vi "Dunk Tank Cal UI.vi"(11 "Calling VI Ref":refnum<vi>) -> ()   [LabVIEW 2013]
uses:
  Netway Driver/Type Defs/Communication Function Type Def.ctl
  <vilib>/ptbypt/NI_PtbyPt.lvlib
  <vilib>/Utility/file.llb/Read From Spreadsheet File (string).vi
  <vilib>/Utility/miscctls.llb/LVRowAndColumnTypeDef.ctl
  <vilib>/Analysis/NI_AALPro.lvlib
  <resource>/objmgr/daqmx.rc
  <vilib>/Utility/file.llb/Write To Spreadsheet File (string).vi
panel:
  in  "App Dir":path
  in  "Load Indicator Tab":enum32{"Page 1"}(tab)
  in  "Header Tab":enum32{"Page 1", "Page 2"}(tab)
  in  "Header OK":bool
  in  "Header Cancel":bool
  in  "Header Comments":string[][](table)=[["PRODUCT 5V. IS REFERENCE ONLY."], ["1"], ["2"]]
  in  "Cal Standards Table":string[][](table)=[["FLUKE MULTIMETER", "3539"], ["FLUKE CALIBRATOR", "7955"], ["", ""], ["", ""], ["", ""]]
  in  "Sys Cal Table":string[][](table)=[["CIB BD.", "DSS 9372-1"], ["D/A BD.", "DSS 9372-2"], ["", ""], ["", ""], ["", ""]]
  in  "Header Table 1":string[][](table)=[["9372blah"], ["DELPHI"], ["TL1181E"], ["EU2C397"], ["CIB/ D/A BD."], ["5 VOLTS"], ["NEW"], ["9087"]]
  in  "Header Table 2":string[][](table)=[["39687"], ["12"], ["40052"], ["MDC"], ["24"], ["48"], ["JUM  /   DR"]]
  in  "debug":bool=TRUE
  in  "Verify Tab":enum32{"Page 1", "Page 2"}(tab)
  in  "Hide Devs":bool
  in  "Auto":bool
  in  "Hide Cal Values":bool
  in  "Verify Edit":bool
  in  "Verify Table":string[][](table)=[["", "0", "0"], ["", "3", "3"], ["", "6", "6"], ["", "9", "9"], ["", "12", "12"], ["", "15", "15"], ["", "", ""], ["", "", ""], ["", "", ""], ["", "", ""]]
  in  "Verify Read":bool
  in  "ms":u32=1000
  in  "avg":i32=5
  in  "Output Tab":enum32{"Page 1", "Page 2"}(tab)
  in  "Close Outputs":bool
  in  "Output Question":bool
  in  "Set Output Next":bool
  in  "Set Output":bool
  in  "Output Listbox":i32(listbox)
  out "Row":i32
  in  "Main Tab":enum32{"Page 1", "Page 2"}(tab)
  in  "View Spreadsheet":bool
  in  "Header":bool
  out "Cal Table":string[][](table)=[["AI-00", "V", "", "", "", "", "", "", "", "", "", "", "", "", "", "", "", "", "", "", "", "", "", "", "", "", "", "", "", "", "", ""], ["AI-01", "V", "", "", "", "", "", "", "", "", "", "", "", "", "", "", "", "", "", "", "", "", "", "", "", "", "", "", "", "", "", ""], ["AI-02", "V", "", "", "", "", "", "", "", "", "", "", "", "", "", "", "", "", "", "", "", "", "", "", "", "", "", "", "", "", "", ""], ["AI-03", "V", "", "", "", "", "", "", "", "", "", "", "", "", "", "", "", "", "", "", "", "", "", "", "", "", "", "", "", "", "", ""], ["AI-04", "V", "", "", "", "", "", "", "", "", "", "", "", "", "", "", "", "", "", "", "", "", "", "", "", "", "", "", "", "", "", ""], ["AI-05", "V", "", "", "", "", "", "", "", "", "", "", "", "", "", "", "", "", "", "", "", "", "", "", "", "", "", "", "", "", "", ""], ["AI-06", "V", "", "", "", "", "", "", "", "", "", "", "", "", "", "", "", "", "", "", "", "", "", "", "", "", "", "", "", "", "", ""], ["AI-07", "V", "", "", "", "", "", "", "", "", "", "", "", "", "", "", "", "", "", "", "", "", "", "", "", "", "", "", "", "", "", ""], ["AI-08", "V", "", "", "", "", "", "", "", "", "", "", "", "", "", "", "", "", "", "", "", "", "", "", "", "", "", "", "", "", "", ""], ["AI-09", "V", "", "", "", "", "", "", "", "", "", "", "", "", "", "", "", "", "", "", "", "", "", "", "", "", "", "", "", "", "", ""], ["AI-10", "V", "", "", "", "", "", "", "", "", "", "", "", "", "", "", "", "", "", "", "", "", "", "", "", "", "", "", "", "", "", ""], ["AI-11", "V", "", "", "", "", "", "", "", "", "", "", "", "", "", "", "", "", "", "", "", "", "", "", "", "", "", "", "", "", "", ""], ["AI-12", "V", "", "", "", "", "", "", "", "", "", "", "", "", "", "", "", "", "", "", "", "", "", "", "", "", "", "", "", "", "", ""], ["AI-13", "V", "", "", "", "", "", "", "", "", "", "", "", "", "", "", "", "", "", "", "", "", "", "", "", "", "", "", "", "", "", ""], ["AI-14", "V", "", "", "", "", "", "", "", "", "", "", "", "", "", "", "", "", "", "", "", "", "", "", "", "", "", "", "", "", "", ""], ["AI-15", "V", "", "", "", "", "", "", "", "", "", "", "", "", "", "", "", "", "", "", "", "", "", "", "", "", "", "", "", "", "", ""], ["AI-16", "V", "", "", "", "", "", "", "", "", "", "", "", "", "", "", "", "", "", "", "", "", "", "", "", "", "", "", "", "", "", ""], ["AI-17", "V", "", "", "", "", "", "", "", "", "", "", "", "", "", "", "", "", "", "", "", "", "", "", "", "", "", "", "", "", "", ""], ["AI-18", "V", "", "", "", "", "", "", "", "", "", "", "", "", "", "", "", "", "", "", "", "", "", "", "", "", "", "", "", "", "", ""], ["AI-19", "V", "", "", "", "", "", "", "", "", "", "", "", "", "", "", "", "", "", "", "", "", "", "", "", "", "", "", "", "", "", ""], ["AI-20", "V", "", "", "", "", "", "", "", "", "", "", "", "", "", "", "", "", "", "", "", "", "", "", "", "", "", "", "", "", "", ""], ["AI-21", "V", "", "", "", "", "", "", "", "", "", "", "", "", "", "", "", "", "", "", "", "", "", "", "", "", "", "", "", "", "", ""], ["AI-22", "V", "", "", "", "", "", "", "", "", "", "", "", "", "", "", "", "", "", "", "", "", "", "", "", "", "", "", "", "", "", ""], ["AI-23", "V", "", "", "", "", "", "", "", "", "", "", "", "", "", "", "", "", "", "", "", "", "", "", "", "", "", "", "", "", "", ""], ["AI-24", "V", "", "", "", "", "", "", "", "", "", "", "", "", "", "", "", "", "", "", "", "", "", "", "", "", "", "", "", "", "", ""], ["AI-25", "V", "", "", "", "", "", "", "", "", "", "", "", "", "", "", "", "", "", "", "", "", "", "", "", "", "", "", "", "", "", ""], ["AI-26", "V", "", "", "", "", "", "", "", "", "", "", "", "", "", "", "", "", "", "", "", "", "", "", "", "", "", "", "", "", "", ""], ["AI-27", "V", "", "", "", "", "", "", "", "", "", "", "", "", "", "", "", "", "", "", "", "", "", "", "", "", "", "", "", "", "", ""], ["AI-28", "V", "", "", "", "", "", "", "", "", "", "", "", "", "", "", "", "", "", "", "", "", "", "", "", "", "", "", "", "", "", ""], ["AI-29", "V", "", "", "", "", "", "", "", "", "", "", "", "", "", "", "", "", "", "", "", "", "", "", "", "", "", "", "", "", "", ""], ["AI-30", "V", "", "", "", "", "", "", "", "", "", "", "", "", "", "", "", "", "", "", "", "", "", "", "", "", "", "", "", "", "", ""], ["AI-31", "V", "", "", "", "", "", "", "", "", "", "", "", "", "", "", "", "", "", "", "", "", "", "", "", "", "", "", "", "", "", ""], ["TC-00", "degF", "", "", "", "", "", "", "", "", "", "", "", "", "", "", "", "", "", "", "", "", "", "", "", "", "", "", "", "", "", ""], ["TC-01", "degF", "", "", "", "", "", "", "", "", "", "", "", "", "", "", "", "", "", "", "", "", "", "", "", "", "", "", "", "", "", ""], ["TC-02", "degF", "", "", "", "", "", "", "", "", "", "", "", "", "", "", "", "", "", "", "", "", "", "", "", "", "", "", "", "", "", ""], ["TC-03", "degF", "", "", "", "", "", "", "", "", "", "", "", "", "", "", "", "", "", "", "", "", "", "", "", "", "", "", "", "", "", ""], ["TC-04", "degF", "", "", "", "", "", "", "", "", "", "", "", "", "", "", "", "", "", "", "", "", "", "", "", "", "", "", "", "", "", ""], ["TC-05", "degF", "", "", "", "", "", "", "", "", "", "", "", "", "", "", "", "", "", "", "", "", "", "", "", "", "", "", "", "", "", ""], ["TC-06", "degF", "", "", "", "", "", "", "", "", "", "", "", "", "", "", "", "", "", "", "", "", "", "", "", "", "", "", "", "", "", ""], ["TC-07", "degF", "", "", "", "", "", "", "", "", "", "", "", "", "", "", "", "", "", "", "", "", "", "", "", "", "", "", "", "", "", ""], ["TC-08", "degF", "", "", "", "", "", "", "", "", "", "", "", "", "", "", "", "", "", "", "", "", "", "", "", "", "", "", "", "", "", ""], ["TC-09", "degF", "", "", "", "", "", "", "", "", "", "", "", "", "", "", "", "", "", "", "", "", "", "", "", "", "", "", "", "", "", ""], ["TC-10", "degF", "", "", "", "", "", "", "", "", "", "", "", "", "", "", "", "", "", "", "", "", "", "", "", "", "", "", "", "", "", ""], ["TC-11", "degF", "", "", "", "", "", "", "", "", "", "", "", "", "", "", "", "", "", "", "", "", "", "", "", "", "", "", "", "", "", ""], ["TC-12", "degF", "", "", "", "", "", "", "", "", "", "", "", "", "", "", "", "", "", "", "", "", "", "", "", "", "", "", "", "", "", ""], ["TC-13", "degF", "", "", "", "", "", "", "", "", "", "", "", "", "", "", "", "", "", "", "", "", "", "", "", "", "", "", "", "", "", ""], ["TC-14", "degF", "", "", "", "", "", "", "", "", "", "", "", "", "", "", "", "", "", "", "", "", "", "", "", "", "", "", "", "", "", ""], ["TC-15", "degF", "", "", "", "", "", "", "", "", "", "", "", "", "", "", "", "", "", "", "", "", "", "", "", "", "", "", "", "", "", ""], ["", "", "", "", "", "", "", "", "", "", "", "", "", "", "", "", "", "", "", "", "", "", "", "", "", "", "", "", "", "", "", ""]]
  out "Dunk Tank":string
  in  "Channel to Cal":u16(ring) items=["AI-00", "AI-01", "AI-02", "AI-03", "AI-04", "AI-05", "AI-06", "AI-07", "AI-16", "AI-17", "AI-18", "AI-19", "AI-20", "AI-21", "AI-22", "AI-23"]
  in  "Start Cal":bool
  in  "Confirm 1st Point":bool
  out "Reading Value 1":dbl caption="reading" format="%#.4g"
  in  "Cal Value 1":dbl caption="cal pt" format="%#.4g"
  in  "Confirm 2nd Point":bool
  out "Reading Value 2":dbl=0.001 caption="reading" format="%#.4g"
  in  "Cal Value 2":dbl caption="cal pt" format="%#.4g"
  in  "Save Cal":bool
  out "f(x)":dbl format="%#.4g"
  out "a0":dbl format="%#.4g"
  out "x":dbl=0.0006000000000000001 format="%#.4g"
  out "a2":dbl format="%#.4g"
  in  "Cancel Cal":bool
  in  "Cal Unit":string
  in  "Confirm 3rd Point":bool
  out "Reading Value 3":dbl=0.0016 caption="reading" format="%#.4g"
  in  "Cal Value 3":dbl caption="cal pt" format="%#.4g"
  out "a1":dbl format="%#.4g"
  out "x2":dbl=0.0006000000000000001 caption="x" format="%#.4g"
  in  "Output Control":bool
  # "System Calibration Components"
  # "Calibration Standards Used"
  # "Output Control"
  # "1) Enter Header Info"
  # "3)  Select Channel to Calibrate"
  # "4) Start Procedure"
  # "5)  Take First Reading"
  # "6)  Take Second Reading"
  # "7)  Take Final Reading"
  # "8)  Review"
  # "9)  Confirm"
  # "Cal Spreadsheet"
  # "*Excel must be closed to return control to this app."
  # "2"
  # "="
  # "+"
  # "+"
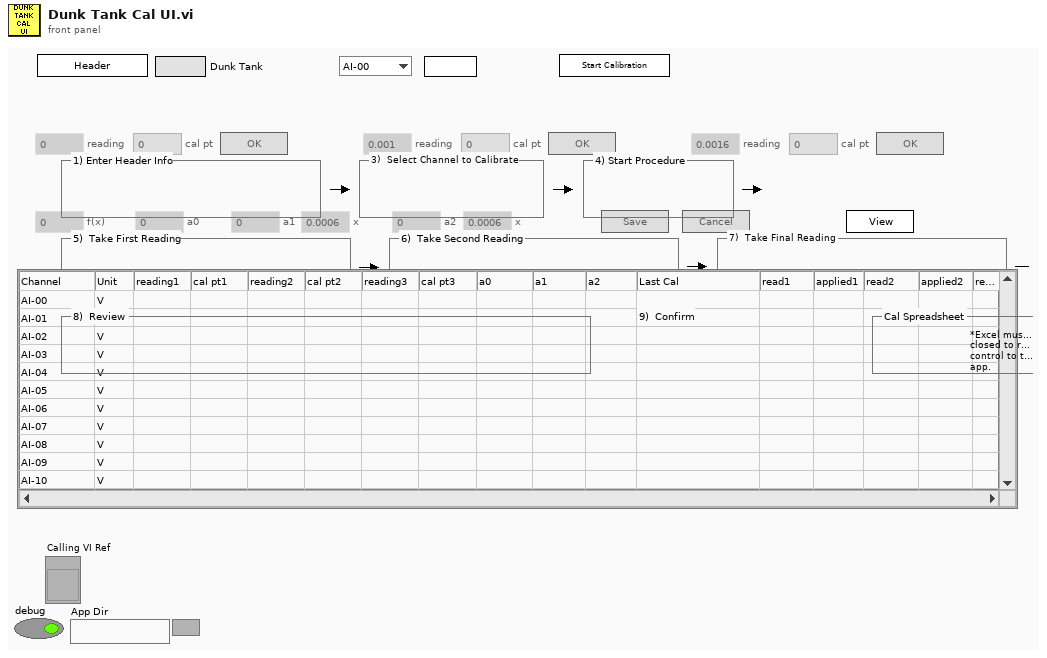
[diagram p1: front panel]
types:
  T1 = cluster{"Error":errorcluster, "Cal Log":string[][], "Cal Log Header":string[], "Cal Files Path":path, "Cal Units":string[], "Default Cal Log":string[][], "AI Targets":string[], "Samples to Avg":i32, "Available Channels":string[], "Output Setpoint":dbl, "Base Path":path, "Cal Targets Path":path, "Calling VI Ref":refnum<vi>, "Dunk Tank SNs":i32[][], "Device":tag, "debug":bool, "Verify Table":string[][], "Cal Template Path":path, "Current Cal Path":path, "Verify Table Ref":refnum<vi>, "Init Mean":bool, "Auto":bool, "App Dir":path, "AI Setpoints":string[]}
  T2 = typedef "Communication Function Type Def.ctl" = enum16{"Find Devices", "Target Device"}
  T3 = enum8{"Enabled", "Disabled", "Disabled and Grayed Out"}
  T4 = typedef "LVRowAndColumnTypeDef.ctl" = cluster{"Row":i32, "Column":i32}
  T5 = enum32{"Bad", "Idle", "Run top level", "Running"}
  T6 = typedef "Registered System.ctl" = cluster{"System Type":T7, "Serial Number":u32, "ID":string, "Cal File?":bool}
  T7 = typedef "System Type.ctl" = enum16{"DAQ Rack", "DAQ Cart", "nx-5000", "unknown", "open"}
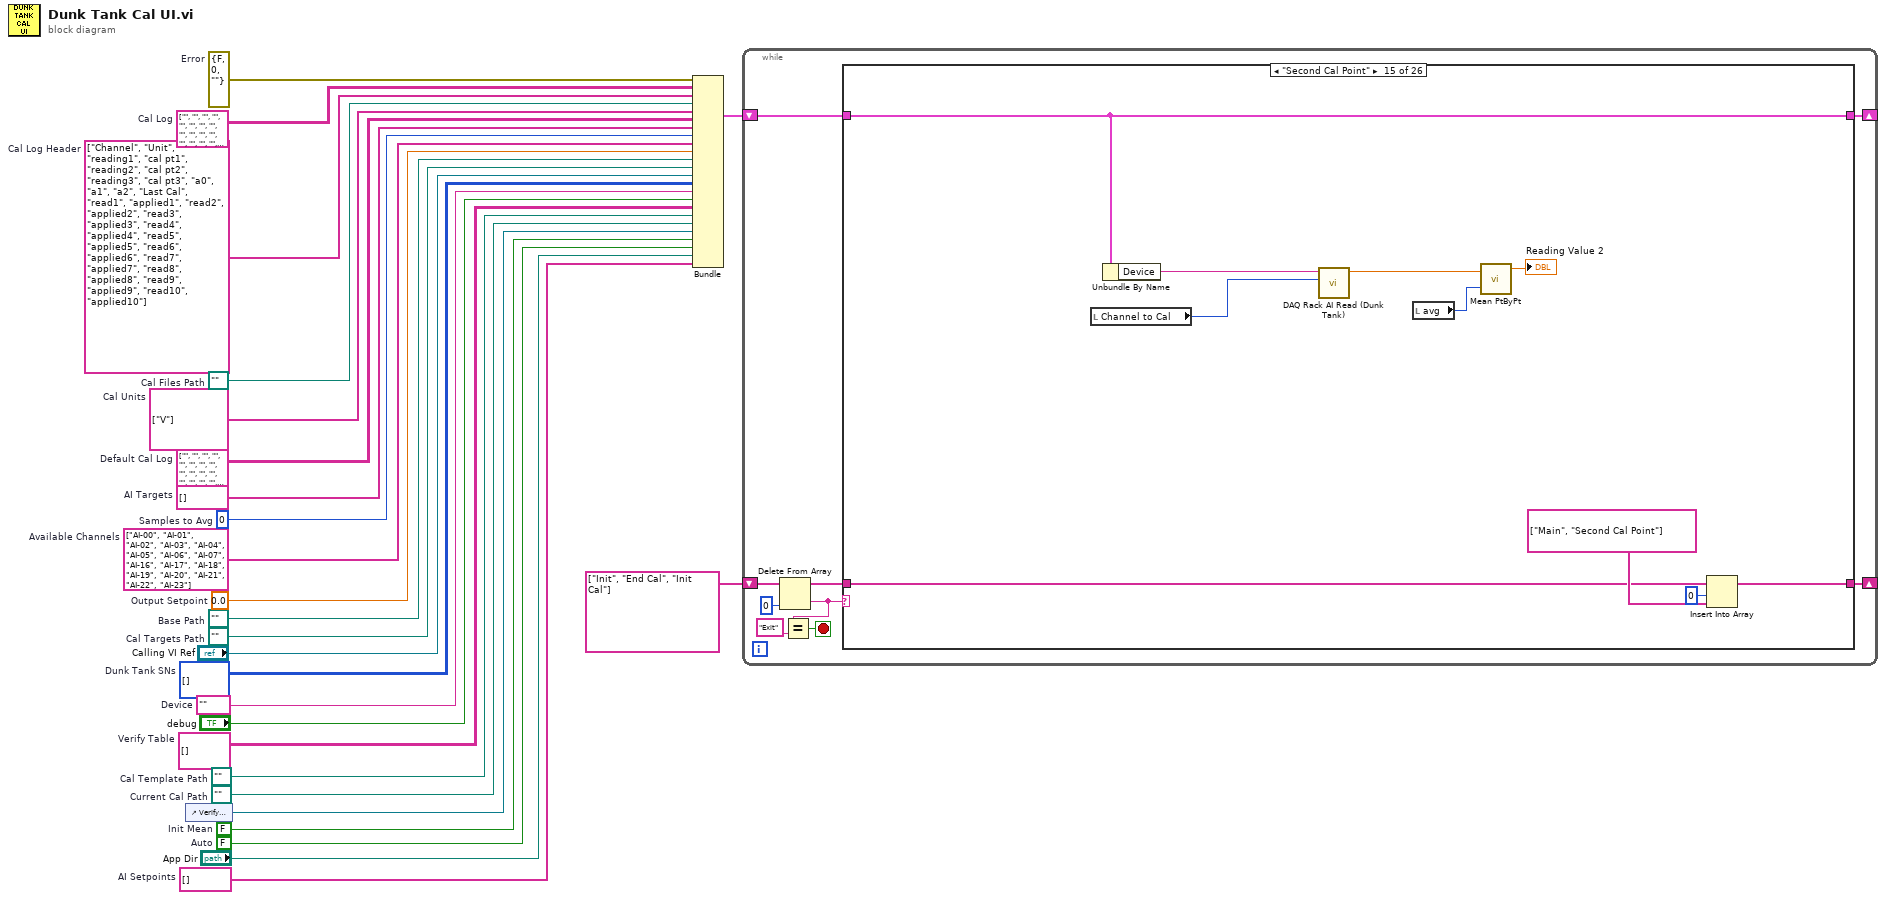
[diagram p0: block diagram]
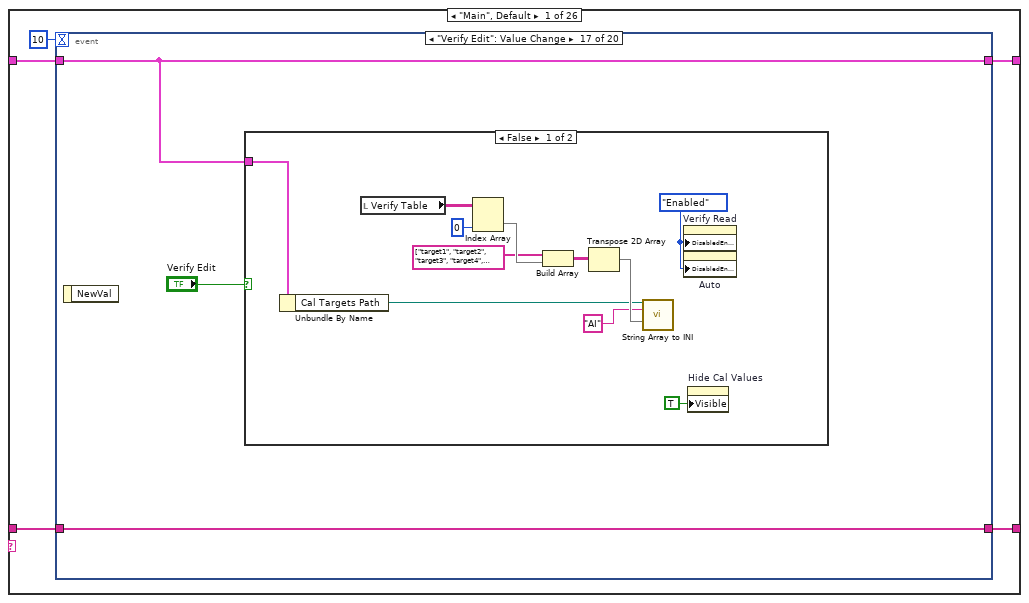
[diagram p2: hidden frame]
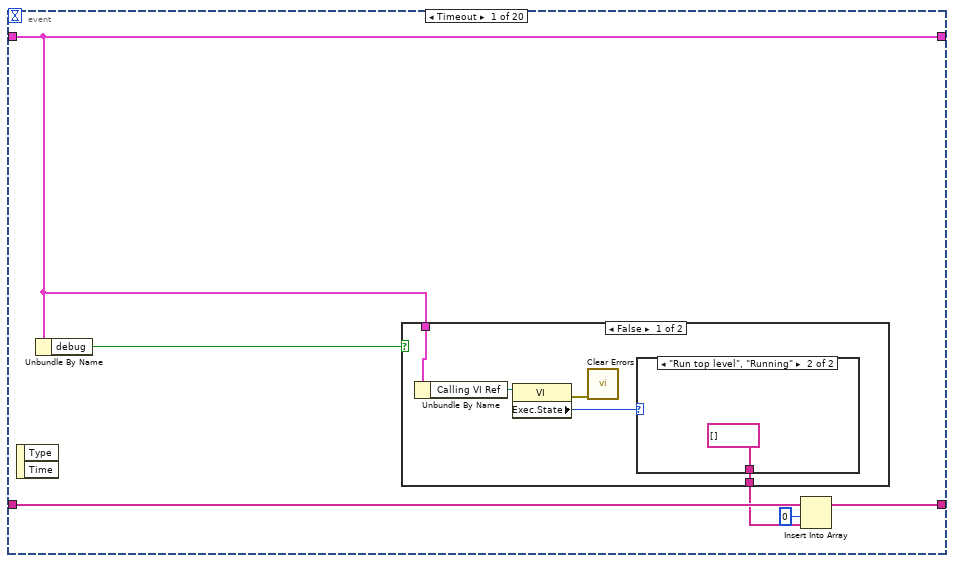
[diagram p3: hidden frame]
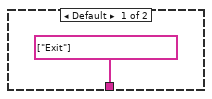
[diagram p4: hidden frame]
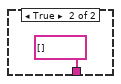
[diagram p5: hidden frame]
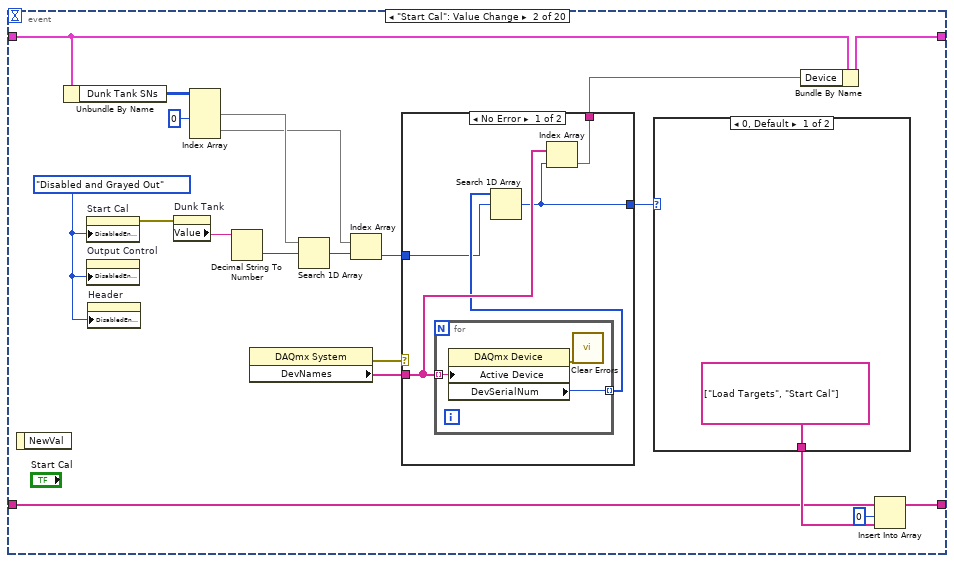
[diagram p6: hidden frame]
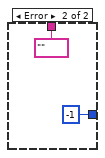
[diagram p7: hidden frame]
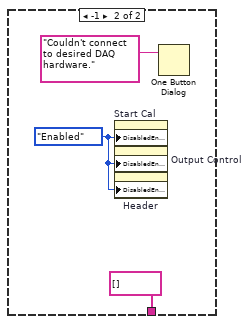
[diagram p8: hidden frame]
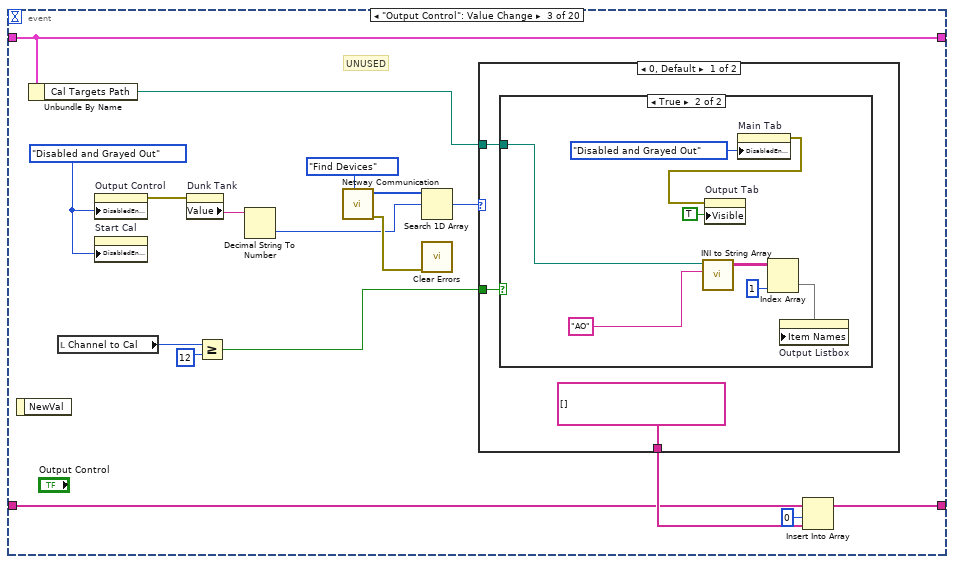
[diagram p9: hidden frame]
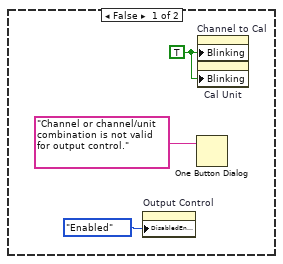
[diagram p10: hidden frame]
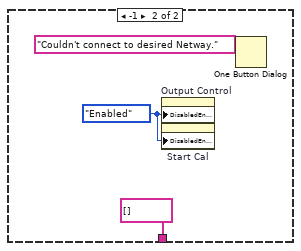
[diagram p11: hidden frame]
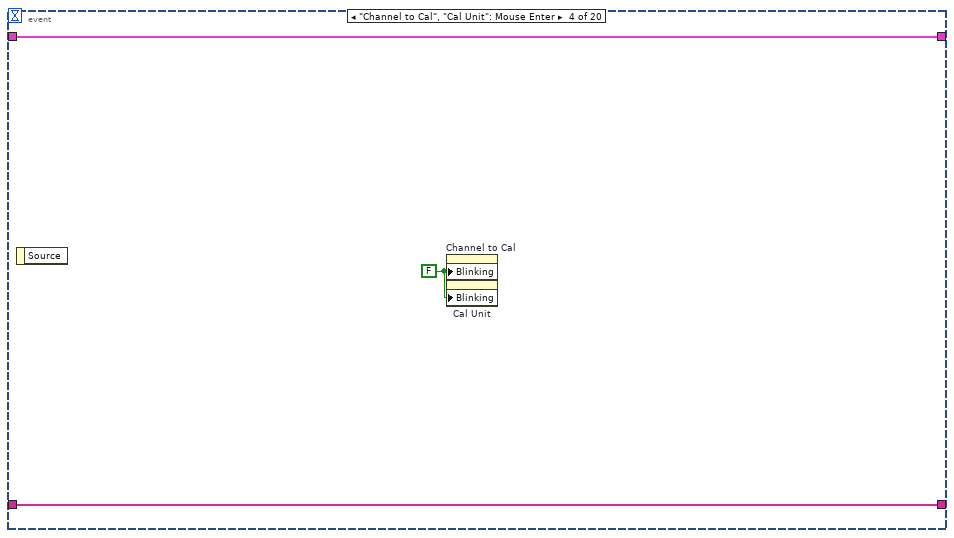
[diagram p12: hidden frame]
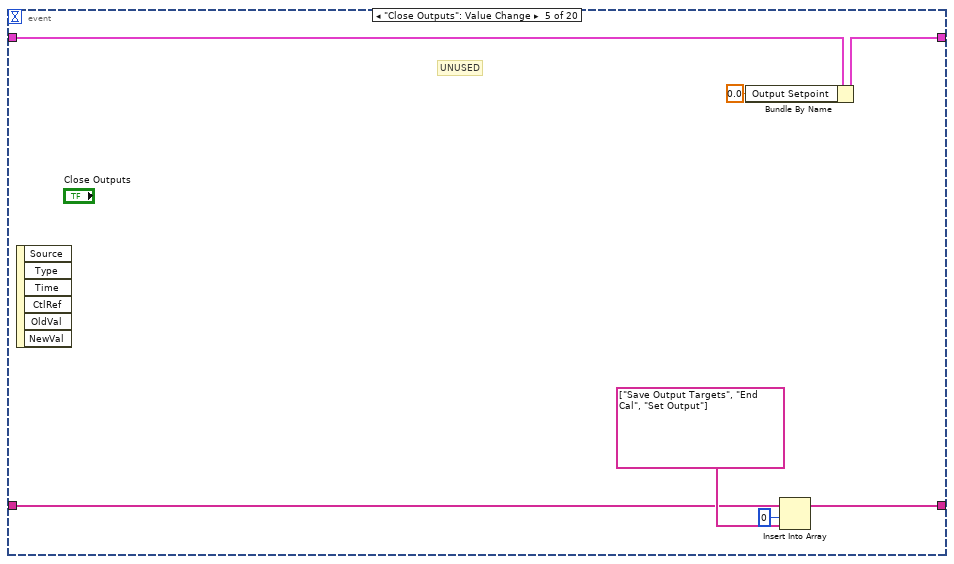
[diagram p13: hidden frame]
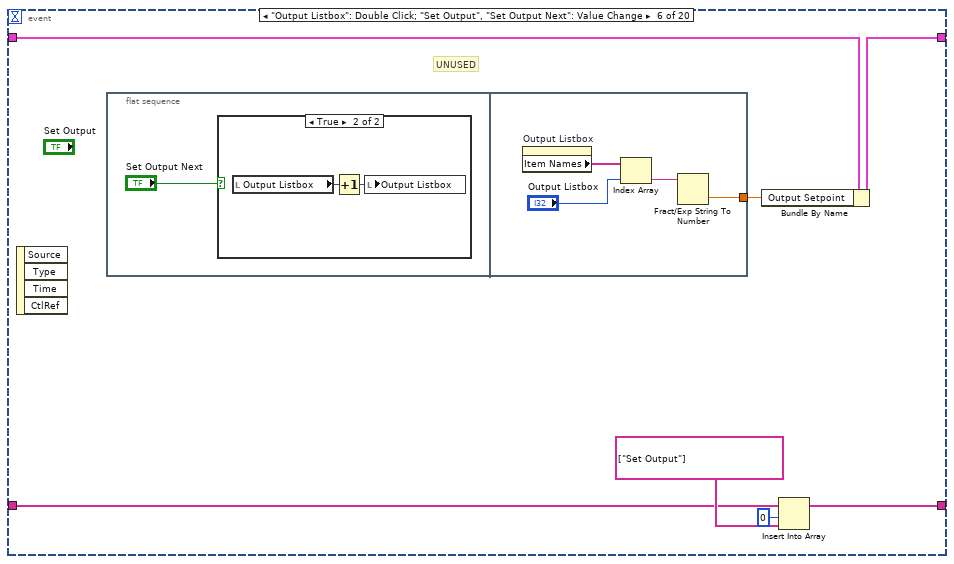
[diagram p14: hidden frame]
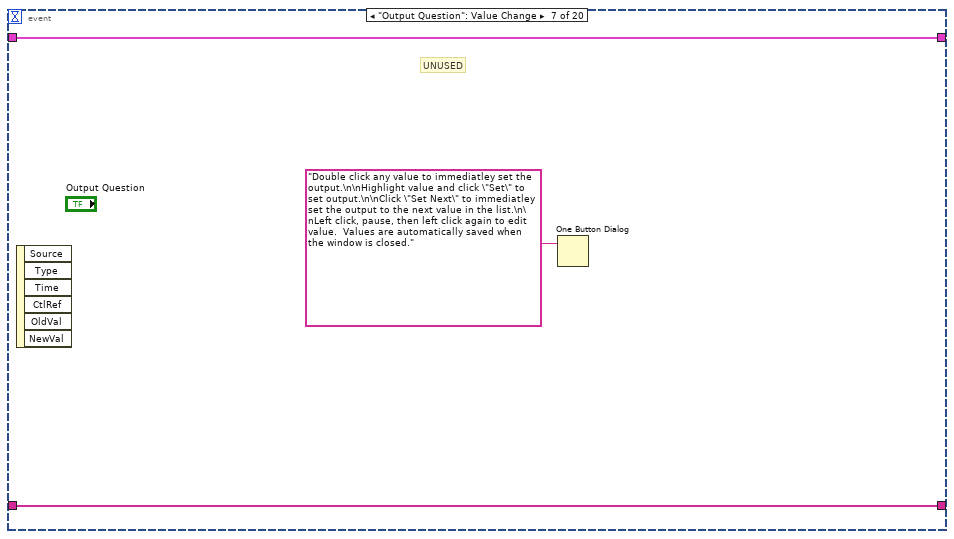
[diagram p16: hidden frame]
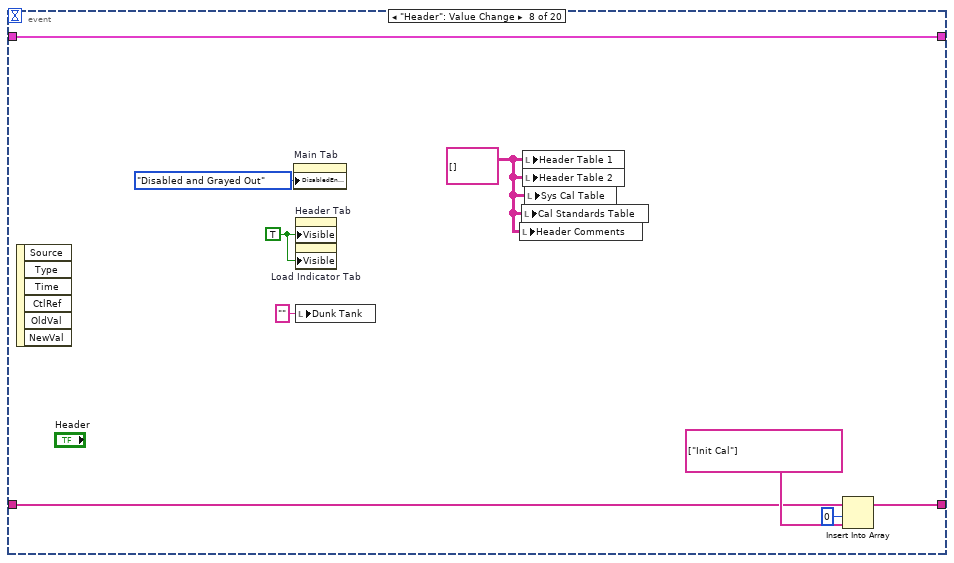
[diagram p17: hidden frame]
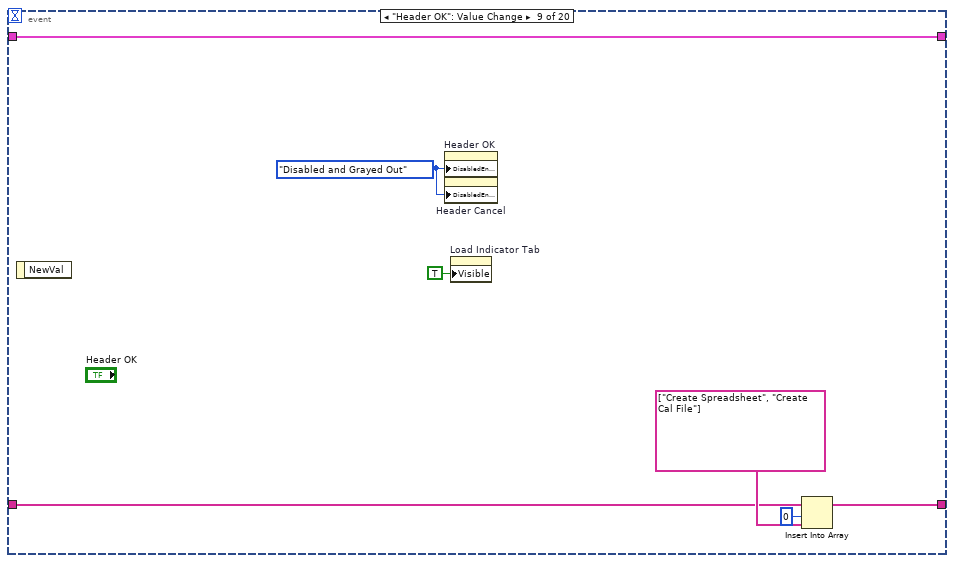
[diagram p18: hidden frame]
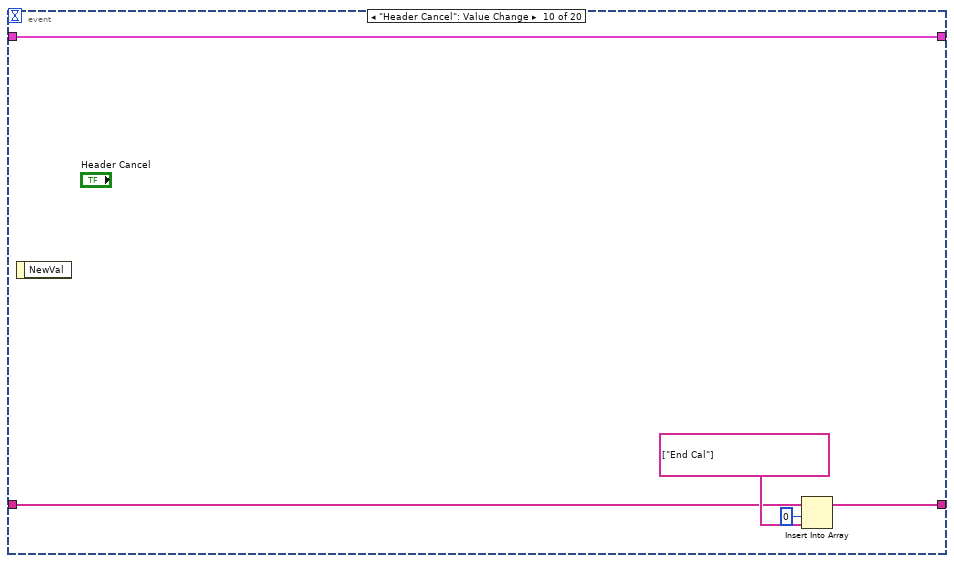
[diagram p19: hidden frame]
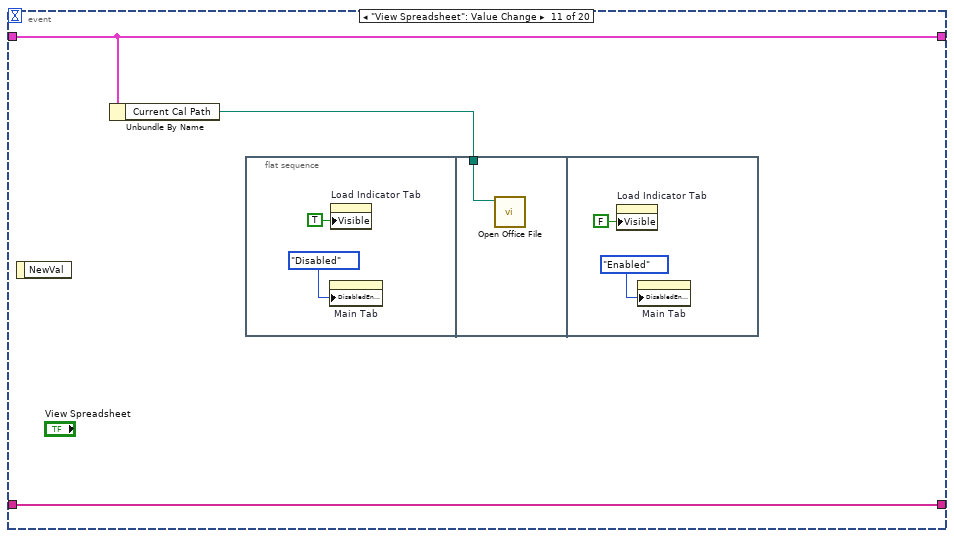
[diagram p20: hidden frame]
diagram:
  w1 = string[] []  # AI Setpoints
  w3 = FALSE  # Auto
  w4 = FALSE  # Init Mean
  w6 = path ""  # Current Cal Path
  w7 = path ""  # Cal Template Path
  w8 = string[][] []  # Verify Table
  w10 = tag ""  # Device
  w11 = i32[][] []  # Dunk Tank SNs
  w13 = path ""  # Cal Targets Path
  w14 = path ""  # Base Path
  w15 = 0.0  # Output Setpoint
  w16 = string[] ["AI-00", "AI-01", "AI-02", "AI-03", "AI-04", "AI-05", "AI-06", "AI-07", "AI-16", "AI-17", "AI-18", "AI-19", "AI-20", "AI-21", "AI-22", "AI-23"]  # Available Channels
  w18 = 0  # Samples to Avg
  w19 = string[] []  # AI Targets
  w20 = string[][] [["", "", "", "", "", "", "", "", "", "", "", "", "", "", "", "", "", "", "", "", "", "", "", "", "", "", "", "", "", "", "", ""], ["", "", "", "", "", "", "", "", "", "", "", "", "", "", "", "", "", "", "", "", "", "", "", "", "", "", "", "", "", "", "", ""], ["", "", "", "", "", "", "", "", "", "", "", "", "", "", "", "", "", "", "", "", "", "", "", "", "", "", "", "", "", "", "", ""], ["", "", "", "", "", "", "", "", "", "", "", "", "", "", "", "", "", "", "", "", "", "", "", "", "", "", "", "", "", "", "", ""], ["", "", "", "", "", "", "", "", "", "", "", "", "", "", "", "", "", "", "", "", "", "", "", "", "", "", "", "", "", "", "", ""], ["", "", "", "", "", "", "", "", "", "", "", "", "", "", "", "", "", "", "", "", "", "", "", "", "", "", "", "", "", "", "", ""], ["", "", "", "", "", "", "", "", "", "", "", "", "", "", "", "", "", "", "", "", "", "", "", "", "", "", "", "", "", "", "", ""], ["", "", "", "", "", "", "", "", "", "", "", "", "", "", "", "", "", "", "", "", "", "", "", "", "", "", "", "", "", "", "", ""], ["", "", "", "", "", "", "", "", "", "", "", "", "", "", "", "", "", "", "", "", "", "", "", "", "", "", "", "", "", "", "", ""], ["", "", "", "", "", "", "", "", "", "", "", "", "", "", "", "", "", "", "", "", "", "", "", "", "", "", "", "", "", "", "", ""], ["", "", "", "", "", "", "", "", "", "", "", "", "", "", "", "", "", "", "", "", "", "", "", "", "", "", "", "", "", "", "", ""], ["", "", "", "", "", "", "", "", "", "", "", "", "", "", "", "", "", "", "", "", "", "", "", "", "", "", "", "", "", "", "", ""], ["", "", "", "", "", "", "", "", "", "", "", "", "", "", "", "", "", "", "", "", "", "", "", "", "", "", "", "", "", "", "", ""], ["", "", "", "", "", "", "", "", "", "", "", "", "", "", "", "", "", "", "", "", "", "", "", "", "", "", "", "", "", "", "", ""], ["", "", "", "", "", "", "", "", "", "", "", "", "", "", "", "", "", "", "", "", "", "", "", "", "", "", "", "", "", "", "", ""], ["", "", "", "", "", "", "", "", "", "", "", "", "", "", "", "", "", "", "", "", "", "", "", "", "", "", "", "", "", "", "", ""]]  # Default Cal Log
  w21 = string[] ["V"]  # Cal Units
  w22 = path ""  # Cal Files Path
  w23 = string[] ["Channel", "Unit", "reading1", "cal pt1", "reading2", "cal pt2", "reading3", "cal pt3", "a0", "a1", "a2", "Last Cal", "read1", "applied1", "read2", "applied2", "read3", "applied3", "read4", "applied4", "read5", "applied5", "read6", "applied6", "read7", "applied7", "read8", "applied8", "read9", "applied9", "read10", "applied10"]  # Cal Log Header
  w24 = string[][] [["", "", "", "", "", "", "", "", "", "", "", "", "", "", "", "", "", "", "", "", "", "", "", "", "", "", "", "", "", "", "", ""], ["", "", "", "", "", "", "", "", "", "", "", "", "", "", "", "", "", "", "", "", "", "", "", "", "", "", "", "", "", "", "", ""], ["", "", "", "", "", "", "", "", "", "", "", "", "", "", "", "", "", "", "", "", "", "", "", "", "", "", "", "", "", "", "", ""], ["", "", "", "", "", "", "", "", "", "", "", "", "", "", "", "", "", "", "", "", "", "", "", "", "", "", "", "", "", "", "", ""], ["", "", "", "", "", "", "", "", "", "", "", "", "", "", "", "", "", "", "", "", "", "", "", "", "", "", "", "", "", "", "", ""], ["", "", "", "", "", "", "", "", "", "", "", "", "", "", "", "", "", "", "", "", "", "", "", "", "", "", "", "", "", "", "", ""], ["", "", "", "", "", "", "", "", "", "", "", "", "", "", "", "", "", "", "", "", "", "", "", "", "", "", "", "", "", "", "", ""], ["", "", "", "", "", "", "", "", "", "", "", "", "", "", "", "", "", "", "", "", "", "", "", "", "", "", "", "", "", "", "", ""], ["", "", "", "", "", "", "", "", "", "", "", "", "", "", "", "", "", "", "", "", "", "", "", "", "", "", "", "", "", "", "", ""], ["", "", "", "", "", "", "", "", "", "", "", "", "", "", "", "", "", "", "", "", "", "", "", "", "", "", "", "", "", "", "", ""], ["", "", "", "", "", "", "", "", "", "", "", "", "", "", "", "", "", "", "", "", "", "", "", "", "", "", "", "", "", "", "", ""], ["", "", "", "", "", "", "", "", "", "", "", "", "", "", "", "", "", "", "", "", "", "", "", "", "", "", "", "", "", "", "", ""], ["", "", "", "", "", "", "", "", "", "", "", "", "", "", "", "", "", "", "", "", "", "", "", "", "", "", "", "", "", "", "", ""], ["", "", "", "", "", "", "", "", "", "", "", "", "", "", "", "", "", "", "", "", "", "", "", "", "", "", "", "", "", "", "", ""], ["", "", "", "", "", "", "", "", "", "", "", "", "", "", "", "", "", "", "", "", "", "", "", "", "", "", "", "", "", "", "", ""], ["", "", "", "", "", "", "", "", "", "", "", "", "", "", "", "", "", "", "", "", "", "", "", "", "", "", "", "", "", "", "", ""]]  # Cal Log
  w17 = errorcluster {"status"=FALSE, "code"=0, "source"=""}  # Error
  n1 = control-ref of="Verify Table Ref"() -> (w5:refnum<vi>)
  n2 = Bundle("Error"=w17, "Cal Log"=w24, "Cal Log Header"=w23, "Cal Files Path"=w22, "Cal Units"=w21, "Default Cal Log"=w20, "AI Targets"=w19, "Samples to Avg"=w18, "Available Channels"=w16, "Output Setpoint"=w15, "Base Path"=w14, "Cal Targets Path"=w13, "Calling VI Ref"="Calling VI Ref", "Dunk Tank SNs"=w11, "Device"=w10, "debug"="debug", "Verify Table"=w8, "Cal Template Path"=w7, "Current Cal Path"=w6, "Verify Table Ref"=w5, "Init Mean"=w4, "Auto"=w3, "App Dir"="App Dir", "AI Setpoints"=w1) -> (w25:T1)  [unwired: 1 in]
  n3 = while {
    shift-right: [w27] -> _
    shift-left: string[] ["Init", "End Cal", "Init Cal"] -> [w35]
    shift-right: [w29] -> _
    shift-left: w25 -> [w30]
    stop <- w34 stop-if-true
    n4 = Delete From Array(array=w35, index=0) -> (deleted portion=w32:string, array with subset deleted=w33:string[])  [unwired: 1 in]
    n5 = Equal?(x=w32, y="Exit" ("x")) -> (x = y?=w34:bool)
    n6 = case shown="\"Second Cal Point\"" w32 {
      tunnel: w33 -> [w39 w275 w281 w291 w324 w327 w331 w357 w397 w425 w444 w489 w500 w511 w521 w531 w554 w593 w647 w658 w669 w692 w707 w715 w745 w750]
      tunnel: w30 -> [w37 w259 w282 w308 w323 w326 w329 w360 w399 w421 w442 w490 w496 w509 w519 w529 w557 w573 w625 w656 w667 w689 w702 w713 w738 w749]
      tunnel: [w36 w278 w282 w307 w322 w326 w329 w359 w399 w421 w446 w483 w496 w509 w519 w529 w557 w568 w625 w655 w667 w689 w702 w713 w738 w749] -> w29
      tunnel: [w38 w275 w281 w305 w324 w327 w330 w358 w398 w426 w445 w489 w501 w512 w520 w530 w555 w594 w648 w657 w668 w692 w708 w715 w745 w750] -> w27
      frame "Main", Default {
        n7 = event shown="[16] \"Verify Edit\": Value Change" {
          selector: _ -> [_ _ _ _ _ _ _ _ _ _ _ _ _ _ _ _ _ _ _ _]
          dyn-events: _ -> [_ _ _ _ _ _ _ _ _ _ _ _ _ _ _ _ _ _ _ _]
          timeout: 10 -> [_ _ _ _ _ _ _ _ _ _ _ _ _ _ _ _ _ _ _ _]
          tunnel: [w46 w73 w101 w124 w131 w138 w148 w152 w161 w168 w173 string[] ["Second Cal Point"] string[] ["Final Cal Point"] string[] ["Calculate Coeffs"] string[] ["End Cal"] w196 w220 w238 w246 string[] ["Calc Dev", "Cal Review"]] -> w38
          tunnel: w39 -> [w45 w72 w102 w124 w130 w137 w148 w153 w160 w169 w173 _ _ _ _ w195 w220 w237 w246 _]
          tunnel: [w43 w62 w96 w125 w127 w136 w149 w158 w165 w167 w171 w180 w186 w192 w193 w198 w222 w240 w244 w253] -> w36
          tunnel: w37 -> [w43 w63 w96 w125 w128 w135 w149 w158 w165 w167 w171 w180 w186 w192 w193 w200 w222 w240 w245 w254]
          event Timeout {
            n8 = event-data() -> ()  [unwired: 1 in, 2 out]
            n9 = Unbundle By Name(w43) -> ("debug"=w42:bool)
            n10 = case shown="False" w42 {
              tunnel: [w51 string[] []] -> w44
              tunnel: w43 -> [w48 _]
              frame False {
                n11 = Unbundle By Name(w48) -> ("Calling VI Ref"=w50:refnum<vi>)
                n12 = property class="VI"(reference=w50) -> (error out=w47:errorcluster, "Exec.State"=w49:T5)  [unwired: 1 in, 1 out]
                n13 = call <vilib>:"Clear Errors.vi"("error in (no error)"=w47) -> ()  [unwired: 6 in, 1 out]
                n14 = case shown="\"Run top level\", \"Running\"" w49 {
                  tunnel: [string[] ["Exit"] string[] []] -> w51
                  frame Default {
                  }
                  frame "Run top level", "Running" {
                  }
                }
              }
              frame True {
              }
            }
            n15 = Insert Into Array(array=w45, index=0, new element=w44) -> (w46:string[])
          }
          event "Start Cal": Value Change {
            w56 = T3."Disabled and Grayed Out" ("Disabled")
            n16 = event-data() -> ()  [unwired: 1 in, 1 out]
            n17 = Unbundle By Name(w63) -> ("Dunk Tank SNs"=w71:i32[][])
            n18 = property on="Start Cal" class="Bool"("DisabledEnum"=w56) -> (error out=w59:errorcluster)  [unwired: 2 in, 1 out]
            n19 = property on="Output Control" class="Bool"("DisabledEnum"=w56) -> ()  [unwired: 2 in, 2 out]
            n20 = property on="Header" class="Bool"("DisabledEnum"=w56) -> ()  [unwired: 2 in, 2 out]
            n21 = property on="Dunk Tank" class="Str"(error in=w59) -> ("Value"=w58:string)  [unwired: 1 in, 2 out]
            n22 = Index Array(array=w71, index (col) #1=0 ("disabled index (col)")) -> (element #1=w69:i32[], element #2=w68:i32[])  [unwired: 3 in]
            n23 = Decimal String To Number(string=w58) -> (number=w55:i32)  [unwired: 2 in, 1 out]
            n24 = property class="DAQmx System"() -> (error out=w60:errorcluster, "DevNames"=w65:tag[])  [unwired: 2 in, 1 out]
            n25 = Search 1D Array(1D array=w69, element=w55) -> (index of element=w67:i32)  [unwired: 1 in]
            n26 = Index Array(array=w68, index=w67) -> (element=w66:i32)
            n27 = case shown="No Error" w60 {
              tunnel: w66 -> [w75 _]
              tunnel: w65 -> [w79 _]
              tunnel: [w78 -1 ("index of element")] -> w64
              tunnel: [w77 tag ""] -> w61
              frame No Error {
                n28 = for {
                  tunnel: w79 -> [w82] mode=indexing
                  tunnel: [w81] -> w76 mode=indexing
                  n29 = property class="DAQmx Device"("Active Device"=w82) -> (error out=w80:errorcluster, "DevSerialNum"=w81:u32)  [unwired: 2 in, 1 out]
                  n30 = call <vilib>:"Clear Errors.vi"("error in (no error)"=w80) -> ()  [unwired: 6 in, 1 out]
                }
                n31 = Search 1D Array(1D array=w76, element=w75) -> (index of element=w78:i32)  [unwired: 1 in]
                n32 = Index Array(array=w79, index=w78) -> (element=w77:tag)
              }
              frame Error {
              }
            }
            n33 = case shown="0, Default" w64 {
              tunnel: [string[] ["Load Targets", "Start Cal"] string[] []] -> w74
              frame 0, Default {
              }
              frame -1 {
                w86 = T3."Enabled" ("Disabled")
                n34 = property on="Start Cal" class="Bool"("DisabledEnum"=w86) -> ()  [unwired: 2 in, 2 out]
                n35 = property on="Output Control" class="Bool"("DisabledEnum"=w86) -> ()  [unwired: 2 in, 2 out]
                n36 = property on="Header" class="Bool"("DisabledEnum"=w86) -> ()  [unwired: 2 in, 2 out]
                n37 = One Button Dialog(message="Couldn't connect to desired DAQ hardware.") -> ()  [unwired: 1 in, 1 out]
              }
            }
            n38 = Bundle By Name(cluster=w63, "Device"=w61) -> (w62:T1)
            n39 = Insert Into Array(array=w72, index=0, new element=w74) -> (w73:string[])
          }
          event "Output Control": Value Change {
            w94 = T3."Disabled and Grayed Out" ("Disabled")
            # "UNUSED"
            n40 = event-data() -> ()  [unwired: 1 in, 1 out]
            n41 = Unbundle By Name(w96) -> ("Cal Targets Path"=w95:path)
            n42 = local read "Channel to Cal"() -> (w97:u16)
            n43 = property on="Output Control" class="Bool"("DisabledEnum"=w94) -> (error out=w92:errorcluster)  [unwired: 2 in, 1 out]
            n44 = property on="Start Cal" class="Bool"("DisabledEnum"=w94) -> ()  [unwired: 2 in, 2 out]
            n45 = property on="Dunk Tank" class="Str"(error in=w92) -> ("Value"=w93:string)  [unwired: 1 in, 2 out]
            n46 = Greater Or Equal?(x=w97, y=u16 12) -> (x >= y?=w89:bool)
            n47 = Decimal String To Number(string=w93) -> (number=w91:i32)  [unwired: 2 in, 1 out]
            n48 = call "Netway Communication.vi"("Function"=Communication_Function_Type_Def."Find Devices") -> ("Error OUT"=w100:errorcluster, "Serial Numbers"=w103:i32[])  [unwired: 7 in, 2 out]
            n49 = Search 1D Array(1D array=w103, element=w91) -> (index of element=w98:i32)  [unwired: 1 in]
            n50 = call <vilib>:"Clear Errors.vi"("error in (no error)"=w100) -> ()  [unwired: 6 in, 1 out]
            n51 = case shown="0, Default" w98 {
              tunnel: [string[] [] string[] []] -> w105
              tunnel: w89 -> [w107 _]
              tunnel: w95 -> [w106 _]
              frame 0, Default {
                n52 = case shown="True" w107 {
                  tunnel: w106 -> [_ w112]
                  frame False {
                    w109 = TRUE ("Blinking")
                    n53 = property on="Output Control" class="Bool"("DisabledEnum"=T3."Enabled" ("Disabled")) -> ()  [unwired: 2 in, 2 out]
                    n54 = One Button Dialog(message="Channel or channel/unit combination is not valid for output control.") -> ()  [unwired: 1 in, 1 out]
                    n55 = property on="Channel to Cal" class="Ring (strict)"("Blinking"=w109) -> ()  [unwired: 2 in, 2 out]
                    n56 = property on="Cal Unit" class="Str"("Blinking"=w109) -> ()  [unwired: 2 in, 2 out]
                  }
                  frame True {
                    n57 = call "INI to String Array.vi"("Section"="AO", "Path"=w112) -> ("Array"=w117:string[][])  [unwired: 8 in, 1 out]
                    n58 = property on="Main Tab" class="TabCtl (strict)"("DisabledEnum"=T3."Disabled and Grayed Out" ("Disabled")) -> (error out=w113:errorcluster)  [unwired: 2 in, 1 out]
                    n59 = property on="Output Tab" class="TabCtl (strict)"(error in=w113, "Visible"=TRUE) -> ()  [unwired: 1 in, 2 out]
                    n60 = Index Array(array=w117, index (col)=1 ("disabled index (col)")) -> (element=w116:string[])  [unwired: 1 in]
                    n61 = property on="Output Listbox" class="LstBox (strict)"("Item Names"=w116) -> ()  [unwired: 2 in, 2 out]
                  }
                }
              }
              frame -1 {
                w120 = T3."Enabled" ("Disabled")
                n62 = property on="Output Control" class="Bool"("DisabledEnum"=w120) -> ()  [unwired: 2 in, 2 out]
                n63 = property on="Start Cal" class="Bool"("DisabledEnum"=w120) -> ()  [unwired: 2 in, 2 out]
                n64 = One Button Dialog(message="Couldn't connect to desired Netway.") -> ()  [unwired: 1 in, 1 out]
              }
            }
            n65 = Insert Into Array(array=w102, index=0, new element=w105) -> (w101:string[])
          }
          event "Channel to Cal", "Cal Unit": Mouse Enter {
            w123 = FALSE ("Blinking")
            n66 = event-data() -> ()  [unwired: 1 in, 1 out]
            n67 = property on="Channel to Cal" class="Ring (strict)"("Blinking"=w123) -> ()  [unwired: 2 in, 2 out]
            n68 = property on="Cal Unit" class="Str"("Blinking"=w123) -> ()  [unwired: 2 in, 2 out]
          }
          event "Close Outputs": Value Change {
            # "UNUSED"
            n69 = event-data() -> ()  [unwired: 1 in, 6 out]
            n70 = Bundle By Name(cluster=w128, "Output Setpoint"=0.0 ("AO Setpoint")) -> (w127:T1)
            n71 = Insert Into Array(array=w130, index=0, new element=string[] ["Save Output Targets", "End Cal", "Set Output"]) -> (w131:string[])
          }
          event "Output Listbox": Double Click; "Set Output", "Set Output Next": Value Change {
            # "UNUSED"
            n72 = event-data() -> ()  [unwired: 1 in, 4 out]
            n73 = flat-sequence {
              tunnel: [w143] -> w134
              frame #0 {
                n74 = case shown="True" "Set Output Next" {
                  frame False {
                  }
                  frame True {
                    n75 = local read "Output Listbox"() -> (w142:i32)
                    n76 = Increment(x=w142) -> (x+1=w141:i32)
                    n77 = local write "Output Listbox"(w141) -> ()
                  }
                }
              }
              frame #1 {
                n78 = property on="Output Listbox" class="LstBox (strict)"() -> ("Item Names"=w146:string[])  [unwired: 2 in, 2 out]
                n79 = Index Array(array=w146, index="Output Listbox") -> (element=w144:string)
                n80 = Fract/Exp String To Number(string=w144) -> (number=w143:dbl)  [unwired: 3 in, 1 out]
              }
            }
            n81 = Bundle By Name(cluster=w135, "Output Setpoint"=w134) -> (w136:T1)
            n82 = Insert Into Array(array=w137, index=0, new element=string[] ["Set Output"]) -> (w138:string[])
          }
          event "Output Question": Value Change {
            # "UNUSED"
            n83 = event-data() -> ()  [unwired: 1 in, 6 out]
            n84 = One Button Dialog(message="Double click any value to immediatley set the output.\n\nHighlight value and click \"Set\" to set output.\n\nClick \"Set Next\" to immediatley set the output to the next value in the list.\n\nLeft click, pause, then left click again to edit value.  Values are automatically saved when the window is closed.") -> ()  [unwired: 1 in, 1 out]
          }
          event "Header": Value Change {
            w156 = string[][] [] ("Header Table 1")
            w155 = TRUE ("Visible")
            n85 = event-data() -> ()  [unwired: 1 in, 6 out]
            n86 = property on="Main Tab" class="TabCtl (strict)"("DisabledEnum"=T3."Disabled and Grayed Out" ("Disabled")) -> ()  [unwired: 2 in, 2 out]
            n87 = property on="Header Tab" class="TabCtl (strict)"("Visible"=w155) -> ()  [unwired: 2 in, 2 out]
            n88 = property on="Load Indicator Tab" class="TabCtl (strict)"("Visible"=w155) -> ()  [unwired: 2 in, 2 out]
            n89 = local write "Dunk Tank"("" ("DAQ Rack")) -> ()
            n90 = local write "Header Comments"(w156) -> ()
            n91 = local write "Cal Standards Table"(w156) -> ()
            n92 = local write "Header Table 1"(w156) -> ()
            n93 = local write "Header Table 2"(w156) -> ()
            n94 = local write "Sys Cal Table"(w156) -> ()
            n95 = Insert Into Array(array=w153, index=0, new element=string[] ["Init Cal"]) -> (w152:string[])
          }
          event "Header OK": Value Change {
            w164 = T3."Disabled and Grayed Out" ("Disabled")
            n96 = event-data() -> ()  [unwired: 1 in, 1 out]
            n97 = property on="Header OK" class="Bool"("DisabledEnum"=w164) -> ()  [unwired: 2 in, 2 out]
            n98 = property on="Header Cancel" class="Bool"("DisabledEnum"=w164) -> ()  [unwired: 2 in, 2 out]
            n99 = property on="Load Indicator Tab" class="TabCtl (strict)"("Visible"=TRUE) -> ()  [unwired: 2 in, 2 out]
            n100 = Insert Into Array(array=w160, index=0, new element=string[] ["Create Spreadsheet", "Create Cal File"]) -> (w161:string[])
          }
          event "Header Cancel": Value Change {
            n101 = event-data() -> ()  [unwired: 1 in, 1 out]
            n102 = Insert Into Array(array=w169, index=0, new element=string[] ["End Cal"]) -> (w168:string[])
          }
          event "View Spreadsheet": Value Change {
            n103 = event-data() -> ()  [unwired: 1 in, 1 out]
            n104 = Unbundle By Name(w171) -> ("Current Cal Path"=w172:path)
            n105 = flat-sequence {
              tunnel: w172 -> [w176]
              frame #0 {
                n106 = property on="Main Tab" class="TabCtl (strict)"("DisabledEnum"=T3."Disabled" ("Disabled")) -> ()  [unwired: 2 in, 2 out]
                n107 = property on="Load Indicator Tab" class="TabCtl (strict)"("Visible"=TRUE) -> ()  [unwired: 2 in, 2 out]
              }
              frame #1 {
                n108 = call "Open Office File.vi"("Selection a Word (.doc, .docx), Excel (.xls, .xlsx), or Powerpoint (.ppt, .pptx) Document..."=w176) -> ()  [unwired: 10 in, 1 out]
              }
              frame #2 {
                n109 = property on="Load Indicator Tab" class="TabCtl (strict)"("Visible"=FALSE) -> ()  [unwired: 2 in, 2 out]
                n110 = property on="Main Tab" class="TabCtl (strict)"("DisabledEnum"=T3."Enabled" ("Disabled")) -> ()  [unwired: 2 in, 2 out]
              }
            }
          }
          event "Confirm 1st Point": Value Change {
            w182 = T3."Disabled and Grayed Out" ("Disabled")
            w183 = T3."Enabled" ("Disabled")
            n111 = event-data() -> ()  [unwired: 1 in, 1 out]
            n112 = property on="Reading Value 1" class="DigNum (strict)"("DisabledEnum"=w182) -> ()  [unwired: 2 in, 2 out]
            n113 = property on="Cal Value 1" class="DigNum (strict)"("DisabledEnum"=w182) -> ()  [unwired: 2 in, 2 out]
            n114 = property on="Confirm 1st Point" class="Bool"("DisabledEnum"=w182) -> ()  [unwired: 2 in, 2 out]
            n115 = property on="Reading Value 2" class="DigNum (strict)"("DisabledEnum"=w183) -> ()  [unwired: 2 in, 2 out]
            n116 = property on="Cal Value 2" class="DigNum (strict)"("DisabledEnum"=w183) -> (error out=w181:errorcluster)  [unwired: 2 in, 1 out]
            n117 = property on="Confirm 2nd Point" class="Bool"("DisabledEnum"=w183) -> ()  [unwired: 2 in, 2 out]
            n118 = property on="Cal Value 2" class="DigNum (strict)"(error in=w181, "Key Focus"=TRUE) -> ()  [unwired: 1 in, 2 out]
          }
          event "Confirm 2nd Point": Value Change {
            w189 = T3."Enabled" ("Disabled")
            w190 = T3."Disabled and Grayed Out" ("Disabled")
            n119 = event-data() -> ()  [unwired: 1 in, 1 out]
            n120 = property on="Reading Value 2" class="DigNum (strict)"("DisabledEnum"=w190) -> ()  [unwired: 2 in, 2 out]
            n121 = property on="Cal Value 2" class="DigNum (strict)"("DisabledEnum"=w190) -> ()  [unwired: 2 in, 2 out]
            n122 = property on="Confirm 2nd Point" class="Bool"("DisabledEnum"=w190) -> ()  [unwired: 2 in, 2 out]
            n123 = property on="Reading Value 3" class="DigNum (strict)"("DisabledEnum"=w189) -> ()  [unwired: 2 in, 2 out]
            n124 = property on="Cal Value 3" class="DigNum (strict)"("DisabledEnum"=w189) -> (error out=w187:errorcluster)  [unwired: 2 in, 1 out]
            n125 = property on="Confirm 3rd Point" class="Bool"("DisabledEnum"=w189) -> ()  [unwired: 2 in, 2 out]
            n126 = property on="Cal Value 3" class="DigNum (strict)"(error in=w187, "Key Focus"=TRUE) -> ()  [unwired: 1 in, 2 out]
          }
          event "Confirm 3rd Point": Value Change {
            n127 = event-data() -> ()  [unwired: 1 in, 1 out]
          }
          event "Cancel Cal": Value Change {
            n128 = event-data() -> ()  [unwired: 1 in, 1 out]
          }
          event "Verify Read": Value Change {
            n129 = event-data() -> ()  [unwired: 1 in, 1 out]
            n130 = case shown="True" "Verify Read" {
              tunnel: [FALSE ("Verify Read") FALSE ("Verify Read")] -> w201
              tunnel: w200 -> [_ _]
              tunnel: w200 -> [w205 w210]
              tunnel: [w205 w209] -> w199
              tunnel: [w203 string[] ["Calc Dev", "Cal Review"]] -> w196
              tunnel: w195 -> [w203 _]
              frame False {
              }
              frame True {
                n131 = local read "Row"() -> (w213:i32)
                n132 = local read "f(x)"() -> (w218:dbl)
                n133 = local read "Verify Table"() -> (w206:string[][])
                n134 = Number To Fractional String(number=w218) -> (F-format string=w212:string)  [unwired: 3 in]
                n135 = Replace Array Subset(array=w206, new element=w212, index (row)=w213, index (col)=1 ("disabled index (col)")) -> (w208:string[][])
                n136 = Increment(x=w213) -> (x+1=w217:i32)
                n137 = Bundle(w217, "disabled index (col)"=1) -> (w214:cluster{i32, "disabled index (col)":i32})  [unwired: 1 in]
                n138 = Bundle By Name(cluster=w210, "Verify Table"=w208) -> (w209:T1)
                n139 = property on="Verify Table" class="Tbl (strict)"("Key Focus"=TRUE, "EditPos"=w214, "Value"=w208) -> ()  [unwired: 2 in, 2 out]
              }
            }
            n140 = local write "Verify Read"(w201) -> ()
            n141 = Bundle By Name(cluster=w199, "Init Mean"=TRUE ("initialize")) -> (w198:T1)
          }
          event "Verify Edit": Value Change {
            n142 = event-data() -> ()  [unwired: 1 in, 1 out]
            n143 = case shown="False" "Verify Edit" {
              tunnel: w222 -> [w226 _]
              frame False {
                w227 = T3."Enabled" ("Disabled")
                n144 = Unbundle By Name(w226) -> ("Cal Targets Path"=w225:path)
                n145 = local read "Verify Table"() -> (w224:string[][])
                n146 = Index Array(array=w224, index (col)=0 ("disabled index (col)")) -> (element=w229:string[])  [unwired: 1 in]
                n147 = Build Array(string[] ["target1", "target2", "target3", "target4", "target5", "target6", "target7", "target8", "target9", "target10"], w229) -> (w231:string[][])
                n148 = Transpose 2D Array(2D array=w231) -> (transposed array=w230:string[][])
                n149 = call "String Array to INI.vi"("Path"=w225, "Section"="AI", "Array"=w230) -> ()  [unwired: 12 in, 1 out]
                n150 = property on="Verify Read" class="Bool (strict)"("DisabledEnum"=w227) -> ()  [unwired: 2 in, 2 out]
                n151 = property on="Auto" class="Bool (strict)"("DisabledEnum"=w227) -> ()  [unwired: 2 in, 2 out]
                n152 = property on="Hide Cal Values" class="Bool"("Visible"=TRUE) -> ()  [unwired: 2 in, 2 out]
              }
              frame True {
                w234 = T3."Disabled and Grayed Out" ("Disabled")
                n153 = property on="Verify Read" class="Bool (strict)"("DisabledEnum"=w234) -> ()  [unwired: 2 in, 2 out]
                n154 = property on="Auto" class="Bool (strict)"("DisabledEnum"=w234) -> ()  [unwired: 2 in, 2 out]
                n155 = property on="Hide Cal Values" class="Bool"("Visible"=FALSE) -> ()  [unwired: 2 in, 2 out]
              }
            }
          }
          event "Save Cal": Value Change {
            n156 = event-data() -> ()  [unwired: 1 in, 1 out]
            n157 = property on="Cal Table" class="Tbl (strict)"("DisabledEnum"=T3."Enabled" ("Disabled")) -> ()  [unwired: 2 in, 2 out]
            n158 = property on="Verify Tab" class="TabCtl (strict)"("Visible"=FALSE) -> ()  [unwired: 2 in, 2 out]
            n159 = Insert Into Array(array=w237, index=0, new element=string[] ["Save Cal"]) -> (w238:string[])
          }
          event "Auto": Value Change {
            n160 = event-data() -> ()  [unwired: 1 in, 1 out]
            n161 = case shown="True" "Auto" {
              frame False {
              }
              frame True {
                n162 = local read "Row"() -> (w247:i32)
                n163 = Bundle("Row"=w247, "disabled index (col)"=1) -> (w248:cluster{"Row":i32, "disabled index (col)":i32})  [unwired: 1 in]
                n164 = property on="Verify Table" class="Tbl (strict)"("Key Focus"=TRUE, "EditPos"=w248) -> ()  [unwired: 2 in, 2 out]
              }
            }
            n165 = Bundle By Name(cluster=w245, "Auto"="Auto") -> (w244:T1)
          }
          event "Verify Table": Value Change {
            n166 = event-data() -> ()  [unwired: 1 in, 1 out]
            n167 = Bundle By Name(cluster=w254, "Verify Table"="Verify Table") -> (w253:T1)
          }
        }
      }
      frame "Init" {
        n168 = Unbundle By Name(w259) -> ("debug"=w258:bool, "App Dir"=w257:path)
        n169 = Select(t=path "C:/Documents and Settings/tzt79f/My Documents/Projects/Calibration Utility", s=w258, f=w257) -> (s? t:f=w256:path)
        n170 = Build Path(base path=w256, name or relative path="App Config.ini") -> (appended path=w269:path)
        n171 = call "Read App Config.vi"("App Config Path"=w269) -> ("Cal Files Path"=w274:path, "Registered Systems"=w271:T6[])  [unwired: 9 in]
        n172 = Build Path(base path=w256, name or relative path="Calibration UIs\\Dunk Tank\\Cal Targets.ini") -> (appended path=w272:path)
        n173 = Build Path(base path=w274, name or relative path="Dunk Tank") -> (appended path=w263:path)
        n174 = Build Path(base path=w263, name or relative path="Dunk Tank Cal Template.xls") -> (appended path=w265:path)
        n175 = Build Path(base path=w256, name or relative path="Calibration UIs\\Dunk Tank\\Dunk Tank Cal Template.xls") -> (appended path=w268:path)
        n176 = Create Folder(path (use dialog)=w263) -> (error out=w276:errorcluster)  [unwired: 2 in, 2 out]
        n177 = call <vilib>:"Clear Errors.vi"("error in (no error)"=w276) -> ("error out"=w261:errorcluster)  [unwired: 6 in]
        n178 = call <vilib>:"Check if File or Folder Exists.vi"("error in (no error)"=w261, "path"=w265) -> ("file or folder exists?"=w266:bool, "dup path"=w267:path)  [unwired: 7 in, 1 out]
        n179 = case shown="False" w266 {
          tunnel: w267 -> [w280 _]
          tunnel: w268 -> [w279 _]
          frame False {
            n180 = Copy(10:w280, 11:w279) -> ()  [unwired: 3 in, 3 out]
          }
          frame True {
          }
        }
        n181 = Bundle By Name(cluster=w259, "Dunk Tank SNs"=w271, "Cal Files Path"=w263, "Base Path"=w256, "Cal Targets Path"=w272, "Cal Template Path"=w265) -> (w278:T1)
        n182 = local write "Dunk Tank"("" ("DAQ Rack")) -> ()
      }
      frame "Unused Items" {
      }
      frame "Init Cal" {
        w295 = FALSE ("Verify Read")
        w297 = T3."Enabled" ("Disabled")
        w296 = T3."Disabled and Grayed Out" ("Disabled")
        w301 = T3."Disabled and Grayed Out" ("Disabled")
        n183 = Unbundle By Name(w308) -> ("Available Channels"=w286:string[], "Default Cal Log"=w285:string[][], "Cal Files Path"=w300:path, "Cal Log Header"=w287:string[])  [unwired: 1 out]
        n184 = local read "Dunk Tank"() -> (w284:string)
        n185 = property on="Verify Read" class="Bool (strict)"("DisabledEnum"=w297) -> ()  [unwired: 2 in, 2 out]
        n186 = property on="Cal Table" class="Tbl (strict)"("DisabledEnum"=w297) -> ()  [unwired: 2 in, 2 out]
        n187 = Empty String/Path?(string/path=w284) -> (empty?=w283:bool)
        n188 = property on="Cal Table" class="Tbl (strict)"("Column Headers[]"=w287) -> ()  [unwired: 2 in, 2 out]
        n189 = local write "Output Listbox"(0 ("AO Listbox")) -> ()
        n190 = case shown="False" w283 {
          tunnel: [w311 w312] -> w306
          tunnel: w286 -> [w310 _]
          tunnel: w285 -> [w309 w312]
          frame False {
            n191 = call "Create Cal File Array (Dunk Tank).vi"("Cal Log IN"=w309, "Available Channels"=w310) -> ("Cal Log OUT"=w311:string[][])  [unwired: 9 in]
            n192 = property on="Channel to Cal" class="Ring (strict)"("Strings []"=w310) -> ()  [unwired: 2 in, 2 out]
          }
          frame True {
          }
        }
        n193 = property on="Save Cal" class="Bool"("DisabledEnum"=w301) -> ()  [unwired: 2 in, 2 out]
        n194 = property on="Cancel Cal" class="Bool (strict)"("DisabledEnum"=w301) -> ()  [unwired: 2 in, 2 out]
        n195 = call <vilib>:"Check if File or Folder Exists.vi"("path"=w300) -> ("file or folder exists?"=w304:bool, "dup path"=w303:path)  [unwired: 8 in, 1 out]
        n196 = case shown="True" w304 {
          tunnel: w303 -> [_ w318]
          tunnel: [string[] [] w317] -> w302
          frame False {
            n197 = One Button Dialog(message="Unable to locate cal files\nfolder.") -> ()  [unwired: 1 in, 1 out]
          }
          frame True {
            n198 = List Folder(path=w318) -> (filenames=w315:string[])  [unwired: 3 in, 3 out]
            n199 = Empty Array?(array=w315) -> (empty?=w316:bool)
            n200 = case shown="False" w316 {
              tunnel: [string[] ["Load Cal File"] string[] []] -> w317
              frame False {
              }
              frame True {
              }
            }
          }
        }
        n201 = Bundle By Name(cluster=w308, "Default Cal Log"=w306, "Auto"=FALSE) -> (w307:T1)
        n202 = local write "Auto"(w295) -> ()
        n203 = local write "Verify Edit"(w295) -> ()
        n204 = property on="Verify Tab" class="TabCtl (strict)"("Visible"=FALSE) -> ()  [unwired: 2 in, 2 out]
        n205 = property on="Hide Cal Values" class="Bool"("Visible"=TRUE) -> ()  [unwired: 2 in, 2 out]
        n206 = local write "Verify Read"(w295) -> ()
        n207 = Insert Into Array(array=w291, index=0, new element=string[] ["Clear Dev Data", "Update Dev Tables", "Load Template"]) -> (w290:string[])
        n208 = property on="Reading Value 1" class="DigNum (strict)"("DisabledEnum"=w296) -> ()  [unwired: 2 in, 2 out]
        n209 = property on="Cal Value 1" class="DigNum (strict)"("DisabledEnum"=w296) -> ()  [unwired: 2 in, 2 out]
        n210 = property on="Confirm 1st Point" class="Bool"("DisabledEnum"=w296) -> ()  [unwired: 2 in, 2 out]
        n211 = property on="Reading Value 2" class="DigNum (strict)"("DisabledEnum"=w296) -> ()  [unwired: 2 in, 2 out]
        n212 = property on="Cal Value 2" class="DigNum (strict)"("DisabledEnum"=w296) -> ()  [unwired: 2 in, 2 out]
        n213 = property on="Confirm 2nd Point" class="Bool"("DisabledEnum"=w296) -> ()  [unwired: 2 in, 2 out]
        n214 = property on="Reading Value 3" class="DigNum (strict)"("DisabledEnum"=w296) -> ()  [unwired: 2 in, 2 out]
        n215 = property on="Cal Value 3" class="DigNum (strict)"("DisabledEnum"=w296) -> ()  [unwired: 2 in, 2 out]
        n216 = property on="Confirm 3rd Point" class="Bool"("DisabledEnum"=w296) -> ()  [unwired: 2 in, 2 out]
        n217 = property on="f(x)" class="DigNum (strict)"("DisabledEnum"=w296) -> ()  [unwired: 2 in, 2 out]
        n218 = property on="a0" class="DigNum (strict)"("DisabledEnum"=w296) -> ()  [unwired: 2 in, 2 out]
        n219 = property on="a1" class="DigNum (strict)"("DisabledEnum"=w296) -> ()  [unwired: 2 in, 2 out]
        n220 = property on="x" class="DigNum (strict)"("DisabledEnum"=w296) -> ()  [unwired: 2 in, 2 out]
        n221 = property on="a2" class="DigNum (strict)"("DisabledEnum"=w296) -> ()  [unwired: 2 in, 2 out]
        n222 = property on="x2" class="DigNum (strict)"("DisabledEnum"=w296) -> ()  [unwired: 2 in, 2 out]
        n223 = Insert Into Array(array=w290, index=0, new element=w302) -> (w305:string[])
      }
      frame "Clear Dev Data" {
        n224 = Bundle By Name(cluster=w323, "Verify Table"=string[][] [["", "", "", "", ""], ["", "", "", "", ""], ["", "", "", "", ""], ["", "", "", "", ""], ["", "", "", "", ""], ["", "", "", "", ""], ["", "", "", "", ""], ["", "", "", "", ""], ["", "", "", "", ""], ["", "", "", "", ""]]) -> (w322:T1)
      }
      frame "Update Dev Tables" {
        n225 = Unbundle By Name(w326) -> ("Verify Table"=w325:string[][])
        n226 = local write "Verify Table"(w325) -> ()
      }
      frame "Load Template" {
        n227 = Unbundle By Name(w329) -> ("Cal Template Path"=w334:path)
        n228 = call <vilib>:"Check if File or Folder Exists.vi"("path"=w334) -> ("file or folder exists?"=w333:bool)  [unwired: 8 in, 2 out]
        n229 = case shown="True" w333 {
          tunnel: [string[] [] string[] []] -> w332
          tunnel: w334 -> [w341 w352]
          tunnel: [FALSE ("Visible") FALSE ("Visible")] -> w335
          tunnel: [w338 w344] -> w336
          tunnel: [w338 w344] -> w337
          frame False {
            w338 = T3."Disabled and Grayed Out" ("Disabled")
            n230 = Format Into String(format string="Can't find cal spreadsheet template!\n\nShould have been here:  \"%s\"" ("message"), w341) -> (resulting string=w340:string)  [unwired: 2 in, 1 out]
            n231 = One Button Dialog(message=w340) -> ()  [unwired: 1 in, 1 out]
          }
          frame True {
            w344 = T3."Enabled" ("Disabled")
            n232 = call "Read Write Header.vi"("Cal Template Path"=w352, "Write (F)"=FALSE) -> ("Header Table 1"=w351:string[][], "Header Table 2"=w350:string[][], "Sys Cal Table"=w347:string[][], "Cal Standards Table"=w346:string[][], "Header Comments"=w348:string[][])  [unwired: 13 in]
            n233 = local write "Header Comments"(w348) -> ()
            n234 = local write "Cal Standards Table"(w346) -> ()
            n235 = local write "Header Table 1"(w351) -> ()
            n236 = local write "Header Table 2"(w350) -> ()
            n237 = local write "Sys Cal Table"(w347) -> ()
          }
        }
        n238 = property on="Load Indicator Tab" class="TabCtl (strict)"("Visible"=w335) -> ()  [unwired: 2 in, 2 out]
        n239 = property on="Header OK" class="Bool"("DisabledEnum"=w336) -> ()  [unwired: 2 in, 2 out]
        n240 = property on="Header Cancel" class="Bool"("DisabledEnum"=w337) -> ()  [unwired: 2 in, 2 out]
        n241 = Insert Into Array(array=w331, index=0, new element=w332) -> (w330:string[])
      }
      frame "Create Spreadsheet" {
        n242 = local read "Header Table 1"() -> (w362:string[][])
        n243 = Unbundle By Name(w360) -> ("Cal Files Path"=w366:path)
        n244 = Index Array(array=w362, index (row)=3, index (col)=0 ("disabled index (col)")) -> (element=w355:string)
        n245 = Format Into String(format string="%s.xls" ("initial string"), w355) -> (resulting string=w368:string)  [unwired: 2 in, 1 out]
        n246 = Build Path(base path=w366, name or relative path=w368) -> (appended path=w369:path)
        n247 = Not A Number/Path/Refnum?(number/path/refnum=w369) -> (NaN/Path/Refnum?=w370:bool)
        n248 = Empty String/Path?(string/path=w355) -> (empty?=w371:bool)
        n249 = Or(x=w370, y=w371) -> (x .or. y?=w372:bool)
        n250 = Build Path(base path=w366, name or relative path="Dunk Tank Cal Template.xls") -> (appended path=w367:path)
        n251 = case shown="False" w372 {
          tunnel: [string[] ["Save Header", "Init Cal"] string[] []] -> w361
          tunnel: w369 -> [w374 _]
          tunnel: w367 -> [w375 _]
          frame False {
            n252 = call <vilib>:"Check if File or Folder Exists.vi"("path"=w374) -> ("file or folder exists?"=w377:bool)  [unwired: 8 in, 2 out]
            n253 = case shown="True" w377 {
              tunnel: [FALSE ("T button?") w381] -> w376
              frame False {
              }
              frame True {
                n254 = Two Button Dialog(message="Cal file already exists.  How do you want to proceed?\n\n\"Use Existing\" will continue with existing file and data.  \"Overwrite\" will destroy all data and start with fresh template", 1:"Overwrite" ("F button name (\"Cancel\")"), 2:"Use Existing" ("T button name (\"OK\")")) -> (T button?=w381:bool)
              }
            }
            n255 = case shown="False" w376 {
              tunnel: w374 -> [w385 _]
              tunnel: w375 -> [w384 _]
              frame False {
                n256 = Copy(9:TRUE ("overwrite (F)"), 10:w385, 11:w384) -> ()  [unwired: 2 in, 3 out]
              }
              frame True {
              }
            }
          }
          frame True {
            w386 = T3."Enabled" ("Disabled")
            n257 = property on="Load Indicator Tab" class="TabCtl (strict)"("Visible"=FALSE) -> ()  [unwired: 2 in, 2 out]
            n258 = property on="Header OK" class="Bool"("DisabledEnum"=w386) -> ()  [unwired: 2 in, 2 out]
            n259 = property on="Header Cancel" class="Bool"("DisabledEnum"=w386) -> ()  [unwired: 2 in, 2 out]
            n260 = One Button Dialog(message="\"Manufacturer Serial #\" is blank or contains invalid characters.") -> ()  [unwired: 1 in, 1 out]
          }
        }
        n261 = Bundle By Name(cluster=w360, "Current Cal Path"=w369) -> (w359:T1)
        n262 = Insert Into Array(array=w357, index=0, new element=w361) -> (w358:string[])
      }
      frame "Save Header" {
        n263 = Unbundle By Name(w399) -> ("Current Cal Path"=w404:path, "Cal Template Path"=w405:path)
        n264 = Build Array(w404, w405) -> (w406:path[])
        n265 = Index Array(array="Header Table 1", index (row)=3, index (col)=0 ("disabled index (col)")) -> (element=→"Dunk Tank":string)
        n266 = for {
          tunnel: "Header Table 2" -> [w414]
          tunnel: "Sys Cal Table" -> [w413]
          tunnel: "Cal Standards Table" -> [w412]
          tunnel: "Header Comments" -> [w411]
          tunnel: [w410] -> w401
          tunnel: "Header Table 1" -> [w408]
          tunnel: w406 -> [w407] mode=indexing
          n267 = call "Read Write Header.vi"("Header Table 1 IN"=w408, "Header Table 2 IN"=w414, "Sys Cal Table IN"=w413, "Cal Standards Table IN"=w412, "Header Comments IN"=w411, "Cal Template Path"=w407, "Write (F)"=TRUE) -> ("Header Table 1"=w410:string[][])  [unwired: 8 in, 4 out]
        }
        n268 = flat-sequence {
          tunnel: w401 -> [_]
          frame #0 {
            w415 = T3."Enabled" ("Disabled")
            w416 = FALSE ("Visible")
            n269 = property on="View Spreadsheet" class="Bool"("DisabledEnum"=w415) -> ()  [unwired: 2 in, 2 out]
            n270 = property on="Main Tab" class="TabCtl (strict)"("DisabledEnum"=w415) -> ()  [unwired: 2 in, 2 out]
            n271 = property on="Dunk Tank" class="Str"("DisabledEnum"=w415) -> ()  [unwired: 2 in, 2 out]
            n272 = property on="Channel to Cal" class="Ring (strict)"("DisabledEnum"=w415) -> ()  [unwired: 2 in, 2 out]
            n273 = property on="Cal Unit" class="Str"("DisabledEnum"=w415) -> ()  [unwired: 2 in, 2 out]
            n274 = property on="Start Cal" class="Bool"("DisabledEnum"=w415) -> ()  [unwired: 2 in, 2 out]
            n275 = property on="Load Indicator Tab" class="TabCtl (strict)"("Visible"=w416) -> ()  [unwired: 2 in, 2 out]
            n276 = property on="Header Tab" class="TabCtl (strict)"("Visible"=w416) -> ()  [unwired: 2 in, 2 out]
          }
        }
        n277 = Insert Into Array(array=w397, index=0, new element=string[] []) -> (w398:string[])
      }
      frame "Create Cal File" {
        n278 = Unbundle By Name(w421) -> ("Cal Files Path"=w420:path, "Cal Log Header"=w424:string[], "Default Cal Log"=w423:string[][])
        n279 = local read "Dunk Tank"() -> (w417:string)
        n280 = Build Array (concatenate)(w424, w423) -> (w422:string[][])
        n281 = Empty String/Path?(string/path=w417) -> (empty?=w418:bool)
        n282 = case shown="False" w418 {
          tunnel: w422 -> [w432 _]
          tunnel: w420 -> [w429 _]
          tunnel: w417 -> [w428 _]
          frame False {
            n283 = Format Into String(format string="%s.cal", w428) -> (resulting string=w430:string)  [unwired: 2 in, 1 out]
            n284 = Build Path(base path=w429, name or relative path=w430) -> (appended path=w435:path)
            n285 = call <vilib>:"Check if File or Folder Exists.vi"("path"=w435) -> ("file or folder exists?"=w434:bool, "dup path"=w433:path)  [unwired: 8 in, 1 out]
            n286 = case shown="False" w434 {
              tunnel: w433 -> [w438 _]
              tunnel: w432 -> [w437 _]
              frame False {
                n287 = call-poly <vilib>:"Write To Spreadsheet File.vi"("delimiter (\\t)"="," ("delimiter (\\t)"), "2D data"=w437, "file path (dialog if empty)"=w438) -> ()  [unwired: 5 in, 1 out]
              }
              frame True {
              }
            }
          }
          frame True {
          }
        }
        n288 = Insert Into Array(array=w425, index=0, new element=string[] ["Load Cal File"]) -> (w426:string[])
      }
      frame "Load Cal File" {
        n289 = Unbundle By Name(w442) -> ("Cal Files Path"=w447:path)
        n290 = local read "Dunk Tank"() -> (w440:string)
        n291 = Empty String/Path?(string/path=w440) -> (empty?=w439:bool)
        n292 = case shown="False" w439 {
          tunnel: w447 -> [w456 _]
          tunnel: [w455 w468] -> w446
          tunnel: [w452 string[] []] -> w443
          tunnel: w442 -> [w449 w468]
          tunnel: w440 -> [w448 _]
          frame False {
            n293 = Format Into String(format string="%s.cal", w448) -> (resulting string=w450:string)  [unwired: 2 in, 1 out]
            n294 = Build Path(base path=w456, name or relative path=w450) -> (appended path=w454:path)
            n295 = call <vilib>:"Check if File or Folder Exists.vi"("path"=w454) -> ("file or folder exists?"=w453:bool)  [unwired: 8 in, 2 out]
            n296 = case shown="True" w453 {
              tunnel: w454 -> [_ w466]
              tunnel: w449 -> [w458 w463]
              tunnel: [w458 w462] -> w455
              tunnel: [string[] ["Create Cal File"] string[] []] -> w452
              frame False {
              }
              frame True {
                n297 = call-poly <vilib>:"Read From Spreadsheet File.vi"("delimiter (\\t)"="," ("delimiter (\\t)"), "file path (dialog if empty)"=w466) -> ("all rows"=w465:string[][])  [unwired: 5 in, 4 out]
                n298 = Delete From Array(array=w465, index (row)=0) -> (array with subset deleted=w459:string[][])  [unwired: 2 in, 1 out]
                n299 = property on="Cal Table" class="Tbl (strict)"("Value"=w459) -> ()  [unwired: 2 in, 2 out]
                n300 = Bundle By Name(cluster=w463, "Cal Log"=w459) -> (w462:T1)
              }
            }
          }
          frame True {
          }
        }
        n301 = Insert Into Array(array=w444, index=0, new element=w443) -> (w445:string[])
      }
      frame "Load Targets" {
        w488 = T3."Disabled and Grayed Out" ("Disabled")
        n302 = Unbundle By Name(w490) -> ("Cal Targets Path"=w469:path, "Verify Table"=w482:string[][])
        n303 = property on="Cal Table" class="Tbl (strict)"("Active Cell"=T4 {"Row"=-2, "Column"=-2} ("Active Cell:Active Cell"), "Cell BG Color"=u32 16448250) -> ()  [unwired: 2 in, 2 out]
        n304 = property on="Dunk Tank" class="Str"("DisabledEnum"=w488) -> ()  [unwired: 2 in, 2 out]
        n305 = property on="Channel to Cal" class="Ring (strict)"("DisabledEnum"=w488) -> ()  [unwired: 2 in, 2 out]
        n306 = property on="Cal Unit" class="Str"("DisabledEnum"=w488) -> ()  [unwired: 2 in, 2 out]
        n307 = property on="Start Cal" class="Bool"("DisabledEnum"=w488) -> ()  [unwired: 2 in, 2 out]
        n308 = property on="Output Control" class="Bool"("DisabledEnum"=w488) -> ()  [unwired: 2 in, 2 out]
        n309 = property on="Cancel Cal" class="Bool (strict)"("DisabledEnum"=T3."Enabled" ("Disabled")) -> ()  [unwired: 2 in, 2 out]
        n310 = call "INI to String Array.vi"("Section"="AI", "Path"=w469) -> ("Array"=w493:string[][])  [unwired: 8 in, 1 out]
        n311 = call "INI to String Array.vi"("Section"="AI Setpoints", "Path"=w469) -> ("Array"=w478:string[][])  [unwired: 8 in, 1 out]
        n312 = Index Array(array=w493, index (col)=1 ("disabled index (col)")) -> (element=w491:string[])  [unwired: 1 in]
        n313 = Index Array(array=w478, index (col)=1 ("disabled index (col)")) -> (element=w476:string[])  [unwired: 1 in]
        n314 = Bundle By Name(cluster=w490, "AI Targets"=w491, "AI Setpoints"=w476) -> (w484:T1)
        n315 = Unbundle By Name(w484) -> ("AI Targets"=w470:string[], "AI Setpoints"=w474:string[])
        n316 = Fract/Exp String To Number(string=w474) -> (number=w475:dbl[])  [unwired: 3 in, 1 out]
        n317 = Index Array(array=w475) -> (element #1=w473:dbl, element #2=w472:dbl, element #3=w471:dbl)  [unwired: 3 in]
        n318 = local write "Cal Value 1"(w473) -> ()
        n319 = local write "Cal Value 2"(w472) -> ()
        n320 = local write "Cal Value 3"(w471) -> ()
        n321 = Replace Array Subset(array=w482, new element=w470, index (col)=0 ("disabled index (col)")) -> (w480:string[][])  [unwired: 1 in]
        n322 = property on="Verify Table" class="Tbl (strict)"("Value"=w480) -> ()  [unwired: 2 in, 2 out]
        n323 = Bundle By Name(cluster=w484, "Verify Table"=w480) -> (w483:T1)
      }
      frame "Start Cal" {
        w497 = T3."Enabled" ("Disabled")
        n324 = property on="Reading Value 1" class="DigNum (strict)"("DisabledEnum"=w497) -> ()  [unwired: 2 in, 2 out]
        n325 = property on="Cal Value 1" class="DigNum (strict)"("DisabledEnum"=w497) -> (error out=w498:errorcluster)  [unwired: 2 in, 1 out]
        n326 = property on="Confirm 1st Point" class="Bool"("DisabledEnum"=w497) -> ()  [unwired: 2 in, 2 out]
        n327 = property on="Cal Value 1" class="DigNum (strict)"(error in=w498, "Key Focus"=TRUE) -> ()  [unwired: 1 in, 2 out]
        n328 = Insert Into Array(array=w500, index=0, new element=string[] ["First Cal Point"]) -> (w501:string[])
      }
      frame "First Cal Point" {
        n329 = local read "Channel to Cal"() -> (w506:u16)
        n330 = Unbundle By Name(w509) -> ("Device"=w507:tag)
        n331 = call "DAQ Rack AI Read (Dunk Tank).vi"("Channel to Cal"=w506, "Device"=w507) -> ("Data"=w505:dbl)  [unwired: 9 in]
        n332 = call <vilib>:"Mean PtByPt.vi"("x"=w505, "sample length"="avg") -> ("mean"=→"Reading Value 1":dbl)  [unwired: 2 in, 1 out]
        n333 = Insert Into Array(array=w511, index=0, new element=string[] ["Main", "First Cal Point"]) -> (w512:string[])
      }
      frame "Second Cal Point" {
        n334 = local read "Channel to Cal"() -> (w516:u16)
        n335 = Unbundle By Name(w519) -> ("Device"=w517:tag)
        n336 = call "DAQ Rack AI Read (Dunk Tank).vi"("Channel to Cal"=w516, "Device"=w517) -> ("Data"=w515:dbl)  [unwired: 9 in]
        n337 = local read "avg"() -> (w513:i32)
        n338 = call <vilib>:"Mean PtByPt.vi"("x"=w515, "sample length"=w513) -> ("mean"=→"Reading Value 2":dbl)  [unwired: 2 in, 1 out]
        n339 = Insert Into Array(array=w521, index=0, new element=string[] ["Main", "Second Cal Point"]) -> (w520:string[])
      }
      frame "Final Cal Point" {
        n340 = local read "Channel to Cal"() -> (w526:u16)
        n341 = Unbundle By Name(w529) -> ("Device"=w527:tag)
        n342 = call "DAQ Rack AI Read (Dunk Tank).vi"("Channel to Cal"=w526, "Device"=w527) -> ("Data"=w525:dbl)  [unwired: 9 in]
        n343 = local read "avg"() -> (w523:i32)
        n344 = call <vilib>:"Mean PtByPt.vi"("x"=w525, "sample length"=w523) -> ("mean"=→"Reading Value 3":dbl)  [unwired: 2 in, 1 out]
        n345 = Insert Into Array(array=w531, index=0, new element=string[] ["Main", "Final Cal Point"]) -> (w530:string[])
      }
      frame "Calculate Coeffs" {
        w544 = T3."Enabled" ("Disabled")
        w549 = T3."Disabled and Grayed Out" ("Disabled")
        n346 = property on="Reading Value 3" class="DigNum (strict)"("DisabledEnum"=w549) -> ()  [unwired: 2 in, 2 out]
        n347 = property on="Cal Value 3" class="DigNum (strict)"("DisabledEnum"=w549) -> ()  [unwired: 2 in, 2 out]
        n348 = property on="Confirm 3rd Point" class="Bool"("DisabledEnum"=w549) -> ()  [unwired: 2 in, 2 out]
        n349 = property on="Cal Table" class="Tbl (strict)"("DisabledEnum"=w549) -> ()  [unwired: 2 in, 2 out]
        n350 = property on="Save Cal" class="Bool"("DisabledEnum"=T3."Enabled" ("Disabled")) -> ()  [unwired: 2 in, 2 out]
        n351 = local read "Reading Value 1"() -> (w539:dbl)
        n352 = local read "Reading Value 2"() -> (w538:dbl)
        n353 = local read "Reading Value 3"() -> (w537:dbl)
        n354 = Build Array("Cal Value 1", "Cal Value 2", "Cal Value 3") -> (w536:dbl[])
        n355 = Build Array(w539, w538, w537) -> (w535:dbl[])
        n356 = property on="Verify Tab" class="TabCtl (strict)"("Visible"=TRUE) -> (error out=w547:errorcluster)  [unwired: 2 in, 1 out]
        n357 = call <vilib>:"General Polynomial Fit Coefficients.vi"("Y"=w536, "polynomial order"=2, "X"=w535) -> ("Polynomial Coefficients"=w534:dbl[])  [unwired: 11 in, 1 out]
        n358 = property on="Verify Table" class="Tbl (strict)"(error in=w547, "Key Focus"=TRUE, "EditPos"=T4 {"Row"=0, "Column"=1} ("Active Cell:Active Cell")) -> ()  [unwired: 1 in, 2 out]
        n359 = Index Array(array=w534) -> (element #1=→"a0":dbl, element #2=→"a1":dbl, element #3=→"a2":dbl)  [unwired: 3 in]
        n360 = Insert Into Array(array=w554, index=0, new element=string[] ["Cal Review"]) -> (w555:string[])
        n361 = property on="f(x)" class="DigNum (strict)"("DisabledEnum"=w544) -> ()  [unwired: 2 in, 2 out]
        n362 = property on="a0" class="DigNum (strict)"("DisabledEnum"=w544) -> ()  [unwired: 2 in, 2 out]
        n363 = property on="a1" class="DigNum (strict)"("DisabledEnum"=w544) -> ()  [unwired: 2 in, 2 out]
        n364 = property on="x" class="DigNum (strict)"("DisabledEnum"=w544) -> ()  [unwired: 2 in, 2 out]
        n365 = property on="a2" class="DigNum (strict)"("DisabledEnum"=w544) -> ()  [unwired: 2 in, 2 out]
        n366 = property on="x2" class="DigNum (strict)"("DisabledEnum"=w544) -> ()  [unwired: 2 in, 2 out]
      }
      frame "Cal Review" {
        n367 = property on="Verify Table" class="Tbl (strict)"() -> ("EditPos"=w591:T4)  [unwired: 2 in, 2 out]
        n368 = Unbundle By Name(w573) -> ("Init Mean"=w574:bool, "Device"=w578:tag, "Auto"=w571:bool, "Verify Table"=w575:string[][])
        n369 = Unbundle(w591) -> ("Row"=w589:i32)  [unwired: 1 out]
        n370 = Greater Or Equal To 0?(x=w589) -> (x >= 0?=w590:bool)
        n371 = Index Array(array=w575, index (row)=w589, index (col)=0 ("disabled index (col)")) -> (element=w581:string)
        n372 = Fract/Exp String To Number(string=w581) -> (number=w565:dbl)  [unwired: 3 in, 1 out]
        n373 = case shown="True" w590 {
          tunnel: w589 -> [_ w597]
          frame False {
          }
          frame True {
            "Row" <- w597
          }
        }
        n374 = local read "Channel to Cal"() -> (w577:u16)
        n375 = Increment(x=w565) -> (x+1=w583:dbl)
        n376 = Empty String/Path?(string/path=w581) -> (empty?=w570:bool)
        n377 = call "DAQ Rack AI Read (Dunk Tank).vi"("Channel to Cal"=w577, "Device"=w578) -> ("Data"=w576:dbl)  [unwired: 9 in]
        n378 = Not(x=w570) -> (.not. x?=w584:bool)
        n379 = local read "avg"() -> (w558:i32)
        n380 = call <vilib>:"Mean PtByPt.vi"("x"=w576, "sample length"=w558, "initialize"=w574) -> ("mean"=w563:dbl)  [unwired: 1 in, 1 out]
        "x" <- w563
        "x2" <- w563
        n381 = local read "a0"() -> (w562:dbl)
        n382 = local read "a1"() -> (w561:dbl)
        n383 = local read "a2"() -> (w560:dbl)
        n384 = Build Array(w562, w561, w560) -> (w559:dbl[])
        n385 = call <vilib>:"1D Polynomial Evaluation PtByPt.vi"("Coefficients: a"=w559, "x"=w563) -> ("y"=w566:dbl)
        "f(x)" <- w566
        n386 = Increment(x=w566) -> (x+1=w582:dbl)
        n387 = Subtract(x=w582, y=w583) -> (x-y=w567:dbl)
        n388 = Divide(x=w567, y=w582) -> (x/y=w587:dbl)
        n389 = Absolute Value(x=w587) -> (abs(x)=w564:dbl)
        n390 = Less?(x=w564, y=0.1) -> (x < y?=w585:bool)
        n391 = Compound Arithmetic op=AND(w571, w585, w584) -> (w580:bool)
        n392 = call "Reading Delay.vi"("Delay"="ms", "In Range"=w580) -> ("Take Reading"=w569:bool)  [unwired: 9 in]
        n393 = case shown="True" w569 {
          selector: w569 -> [_ w596]
          frame False {
          }
          frame True {
            n394 = property on="Verify Read" class="Bool (strict)"("Val(Sgnl)"=w596) -> ()  [unwired: 2 in, 2 out]
          }
        }
        n395 = Insert Into Array(array=w593, index=0, new element=string[] ["Main", "Cal Review"]) -> (w594:string[])
        n396 = Bundle By Name(cluster=w573, "Init Mean"=FALSE) -> (w568:T1)
      }
      frame "Save Cal" {
        w620 = u16 4 ("y")
        n397 = Unbundle By Name(w625) -> ("Cal Files Path"=w636:path, "Cal Log Header"=w628:string[], "Cal Log"=w634:string[][], "Verify Table"=w600:string[][])
        n398 = local read "Reading Value 1"() -> (w646:dbl)
        n399 = local read "Reading Value 2"() -> (w644:dbl)
        n400 = local read "Reading Value 3"() -> (w607:dbl)
        n401 = local read "Cal Value 1"() -> (w645:dbl)
        n402 = local read "Cal Value 2"() -> (w643:dbl)
        n403 = local read "Cal Value 3"() -> (w606:dbl)
        n404 = property on="Channel to Cal" class="Ring (strict)"() -> ("RingText.Text"=w635:string)  [unwired: 2 in, 2 out]
        n405 = local read "Dunk Tank"() -> (w602:string)
        n406 = local read "a0"() -> (w605:dbl)
        n407 = local read "a1"() -> (w604:dbl)
        n408 = local read "a2"() -> (w603:dbl)
        n409 = Format Date/Time String(time format string (%c)="%d%b%y %I:%M:%S %p") -> (date/time string=w639:string)  [unwired: 2 in]
        n410 = Index Array(array=w600, index (col) #1=0 ("disabled index (col)"), index (col) #2=1 ("disabled index (col)")) -> (element #1=w610:string[], element #2=w609:string[])  [unwired: 2 in]
        n411 = Format Into String(format string="%s.cal", w602) -> (resulting string=w629:string)  [unwired: 2 in, 1 out]
        n412 = Build Array(w646, w645, w644, w643, w607, w606, w605, w604, w603) -> (w642:dbl[])
        n413 = Interleave 1D Arrays(w610, w609) -> (w608:string[])
        n414 = To Upper Case(1:w639) -> (0:w637:string)
        n415 = Number To Fractional String(number=w642, precision (6)=i16 4) -> (F-format string=w640:string[])  [unwired: 2 in]
        n416 = Build Path(base path=w636, name or relative path=w629) -> (appended path=w630:path)
        n417 = Build Array (concatenate)(w635, "Cal Unit", w640, w637, w608) -> (w633:string[])
        n418 = Replace Array Subset(array=w634, new element=w633, index (row)="Channel to Cal") -> (w627:string[][])  [unwired: 1 in]
        n419 = Build Array (concatenate)(w628, w627) -> (w626:string[][])
        n420 = Bundle(cluster=T4 {"Row"=0, "Column"=0} ("Active Cell:Active Cell"), "Row"="Channel to Cal", "Column"=-2) -> (w621:T4)
        n421 = Greater?(x="Channel to Cal", y=w620) -> (0:w619:bool)
        n422 = Subtract(x="Channel to Cal", y=w620) -> (x-y=w618:u16)
        n423 = call-poly <vilib>:"Write To Spreadsheet File.vi"("delimiter (\\t)"="," ("delimiter (\\t)"), "2D data"=w626, "file path (dialog if empty)"=w630) -> ()  [unwired: 5 in, 1 out]
        n424 = Select(t=w618, s=w619, f=u16 0 ("y")) -> (s? t:f=w615:u16)
        n425 = Bundle(cluster=T4 {"Row"=0, "Column"=0} ("Active Cell:Active Cell"), "Row"=w615, "Column"=0) -> (w614:T4)
        n426 = Insert Into Array(array=w647, index=0, new element=string[] ["Write to Excel", "Load Cal File", "End Cal"]) -> (w648:string[])
        n427 = property on="Cal Table" class="Tbl (strict)"("Active Cell"=w621, "Cell BG Color"=u32 16775793, "Index Values"=w614) -> ()  [unwired: 2 in, 2 out]
      }
      frame "Calc Dev" {
        n428 = Unbundle By Name(w656) -> ("Verify Table"=w653:string[][], "Verify Table Ref"=w652:refnum<vi>)
        n429 = local read "Cal Unit"() -> (w650:string)
        n430 = call "Calc Dev (DAQ Rack).vi"("Verify Table IN"=w653, "Units"=w650, "Dev Table 1 Ref"=w652) -> ("Verify Table OUT"=w651:string[][])  [unwired: 16 in]
        n431 = local write "Verify Table"(w651) -> ()
        n432 = Bundle By Name(cluster=w656, "Verify Table"=w651) -> (w655:T1)
        n433 = Insert Into Array(array=w658, index=0, new element=string[] []) -> (w657:string[])
      }
      frame "Write to Excel" {
        n434 = Unbundle By Name(w667) -> ("Current Cal Path"=w671:path, "Verify Table"=w664:string[][])
        n435 = property on="Channel to Cal" class="Ring (strict)"() -> ("RingText.Text"=w662:string)  [unwired: 2 in, 2 out]
        n436 = local read "Cal Unit"() -> (w660:string)
        n437 = flat-sequence {
          tunnel: w671 -> [w678]
          tunnel: [w678] -> w672
          tunnel: [w675] -> w665
          tunnel: w664 -> [w675]
          tunnel: [w674] -> w663
          tunnel: w662 -> [w674]
          tunnel: [w673] -> w661
          tunnel: w660 -> [w673]
          tunnel: w672 -> [w682]
          tunnel: w665 -> [w681]
          tunnel: w663 -> [w680]
          tunnel: w661 -> [w679]
          frame #0 {
            n438 = property on="Main Tab" class="TabCtl (strict)"("DisabledEnum"=T3."Disabled" ("Disabled")) -> ()  [unwired: 2 in, 2 out]
            n439 = property on="Load Indicator Tab" class="TabCtl (strict)"("Visible"=TRUE) -> ()  [unwired: 2 in, 2 out]
          }
          frame #1 {
            n440 = call "Write DAQ Rack Data.vi"("Cal Unit"=w679, "Channel"=w680, "Verify Table"=w681, "Cal Path"=w682) -> ()  [unwired: 8 in]
          }
          frame #2 {
            n441 = property on="Main Tab" class="TabCtl (strict)"("DisabledEnum"=T3."Enabled" ("Disabled")) -> ()  [unwired: 2 in, 2 out]
            n442 = property on="Load Indicator Tab" class="TabCtl (strict)"("Visible"=FALSE) -> ()  [unwired: 2 in, 2 out]
          }
        }
        n443 = Insert Into Array(array=w669, index=0, new element=string[] ["Recolor Tables"]) -> (w668:string[])
      }
      frame "Recolor Tables" {
        n444 = Unbundle By Name(w689) -> ("Verify Table Ref"=w688:refnum<vi>)
        n445 = property on="Property Node" class="Tbl (strict)"(reference=w688, "Active Cell"=T4 {"Row"=-2, "Column"=-2} ("Active Cell:Active Cell"), "Cell BG Color"=u32 15527148) -> (reference out=w685:refnum<vi>)  [unwired: 1 in, 1 out]
        n446 = property on="Property Node" class="Tbl (strict)"(reference=w685, "Active Cell"=T4 {"Row"=-2, "Column"=1} ("Active Cell:Active Cell"), "Cell BG Color"=u32 16448250) -> ()  [unwired: 1 in, 2 out]
      }
      frame "End Cal" {
        w703 = T3."Disabled and Grayed Out" ("Disabled")
        w704 = 0.0 ("Reading Value 1")
        w696 = FALSE ("Visible")
        n447 = Unbundle By Name(w702) -> ("Current Cal Path"=w701:path)
        n448 = Empty String/Path?(string/path=w701) -> (empty?=w700:bool)
        n449 = property on="Output Tab" class="TabCtl (strict)"("Visible"=w696) -> ()  [unwired: 2 in, 2 out]
        n450 = property on="Header Tab" class="TabCtl (strict)"("Visible"=w696) -> ()  [unwired: 2 in, 2 out]
        n451 = property on="Load Indicator Tab" class="TabCtl (strict)"("Visible"=w696) -> ()  [unwired: 2 in, 2 out]
        n452 = property on="Cancel Cal" class="Bool (strict)"("Value"=FALSE ("Cancel Cal")) -> ()  [unwired: 2 in, 2 out]
        n453 = Select(t=2, s=w700, f=0) -> (s? t:f=w697:i32)
        n454 = property on="Main Tab" class="TabCtl (strict)"("DisabledEnum"=T3."Enabled" ("Disabled")) -> ()  [unwired: 2 in, 2 out]
        n455 = property on="Dunk Tank" class="Str"("DisabledEnum"=w697) -> ()  [unwired: 2 in, 2 out]
        n456 = property on="Channel to Cal" class="Ring (strict)"("DisabledEnum"=w697) -> ()  [unwired: 2 in, 2 out]
        n457 = property on="Start Cal" class="Bool"("DisabledEnum"=w697) -> ()  [unwired: 2 in, 2 out]
        n458 = property on="Cal Unit" class="Str"("DisabledEnum"=w697) -> ()  [unwired: 2 in, 2 out]
        n459 = property on="Output Control" class="Bool"("DisabledEnum"=w697) -> ()  [unwired: 2 in, 2 out]
        n460 = property on="View Spreadsheet" class="Bool"("DisabledEnum"=w697) -> ()  [unwired: 2 in, 2 out]
        n461 = property on="Header" class="Bool"("DisabledEnum"=T3."Enabled" ("Disabled")) -> ()  [unwired: 2 in, 2 out]
        n462 = local write "Reading Value 1"(w704) -> ()
        n463 = local write "Reading Value 2"(w704) -> ()
        n464 = local write "Reading Value 3"(w704) -> ()
        n465 = local write "Cal Value 1"(w704) -> ()
        n466 = local write "Cal Value 2"(w704) -> ()
        n467 = local write "Cal Value 3"(w704) -> ()
        n468 = local write "a0"(w704) -> ()
        n469 = local write "a1"(w704) -> ()
        n470 = local write "a2"(w704) -> ()
        n471 = property on="Header OK" class="Bool"("DisabledEnum"=w703) -> ()  [unwired: 2 in, 2 out]
        n472 = property on="Header Cancel" class="Bool"("DisabledEnum"=w703) -> ()  [unwired: 2 in, 2 out]
        n473 = Insert Into Array(array=w707, index=0, new element=string[] ["Recolor Tables", "Init Cal"]) -> (w708:string[])
      }
      frame "Set Output" {
        # "UNUSED"
        n474 = Unbundle By Name(w713) -> ("Output Setpoint"=w712:dbl)
        n475 = local read "Dunk Tank"() -> (w709:string)
        n476 = local read "Channel to Cal"() -> (w710:u16)
        n477 = Decimal String To Number(string=w709) -> (number=w714:i32)  [unwired: 2 in, 1 out]
        n478 = local read "Cal Unit"() -> (w711:string)
        n479 = case shown="\"1\"" w711 {
          tunnel: w714 -> [w723 w729 w736]
          tunnel: w712 -> [w722 w726 w733]
          tunnel: w710 -> [w718 w728 w735]
          frame "0", Default {
            n480 = Multiply(x=w722, y=1000.0) -> (x*y=w720:dbl)
            n481 = Subtract(x=w718, y=u16 11) -> (x-y=w716:u16)
            n482 = To Long Integer(number=w720) -> (32bit integer=w719:i32)
            n483 = call "Write Analog Outputs.vi"("Value"=w719, "Analog Output"=w716, "Serial Number"=w723) -> ()  [unwired: 8 in, 1 out]
          }
          frame "1" {
            n484 = Increment(x=w728) -> (x+1=w727:u16)
            n485 = To Long Integer(number=w726) -> (32bit integer=w725:i32)
            n486 = case shown="0" w725 {
              tunnel: [1000 ("Frequency") 0 ("Frequency")] -> w724
              frame Default {
              }
              frame 0 {
              }
            }
            n487 = call "Write Pwm Outputs.vi"("Serial Number"=w729, "Output"=w727, "Duty"=w725, "Frequency"=w724) -> ()  [unwired: 11 in, 1 out]
          }
          frame "2" {
            n488 = Increment(x=w735) -> (x+1=w734:u16)
            n489 = call "Write Pwm Outputs.vi"("Serial Number"=w736, "Output"=w734, "Duty"=50 ("Frequency"), "Frequency"=w733) -> ()  [unwired: 11 in, 1 out]
          }
        }
      }
      frame "Save Output Targets" {
        # "UNUSED"
        n490 = Unbundle By Name(w738) -> ("Cal Targets Path"=w737:path)
        n491 = local read "Cal Unit"() -> (w740:string)
        n492 = property on="Output Listbox" class="LstBox (strict)"() -> ("Item Names"=w741:string[])  [unwired: 2 in, 2 out]
        n493 = case shown="\"0\", Default" w740 {
          tunnel: ["AO" ("Section") "%_out" ("Section") "Hz_out" ("Section")] -> w739
          frame "0", Default {
          }
          frame "1" {
          }
          frame "2" {
          }
        }
        n494 = Build Array(string[] ["target1", "target2", "target3", "target4", "target5", "target6", "target7", "target8", "target9", "target10"], w741) -> (w744:string[][])
        n495 = Transpose 2D Array(2D array=w744) -> (transposed array=w743:string[][])
        n496 = call "String Array to INI.vi"("Path"=w737, "Section"=w739, "Array"=w743) -> ()  [unwired: 12 in, 1 out]
      }
      frame "Exit" {
      }
    }
  }
